vi "OOB Performance Test varaiable.vi"() -> ()   [LabVIEW 2021]
uses:
  <vilib>/Platform/TimedLoop/XDataNode/timing_clust.ctl
  <vilib>/Platform/TimedLoop/XDataNode/nitl_modes.ctl
  <vilib>/Platform/TimedLoop/XDataNode/wakeup.ctl
  CIFOutOfBand.lvclass/CIFOutOfBand.ctl
  CIFCore/Common/Typedef/Plugin Status.ctl
  CIFCore/Common/Typedef/Plugin State.ctl
  CIFCore/Common/Typedef/Timing Statistics.ctl
  CIFCore/Common/Typedef/Timing Stats Base.ctl
  CIFCore/Common/Typedef/FIFO Statistics.ctl
  CIFCore/Common/Typedef/Simple Error.ctl
  CIFCore/Common/Typedef/Monitor Doubles.ctl
  CIFCore/Common/Typedef/Monitor U64.ctl
  CIFCore/Common/Typedef/Monitor I64.ctl
  CIFOutOfBand.lvclass
  <vilib>/Platform/TimedLoop/XDataNode/XDataNode.xnode
  <vilib>/Platform/TimedLoop/XDataNode/XDNodeRunTimeDep.lvlib
  CIFCore/Common/CIFCoreCommon.lvlib
panel:
  out "avg complexwrite":dbl
  out "Max Complexwrite":dbl
  out "avg complexnote write":dbl
  out "Max Complexnote write":dbl
  out "avg complexnote":dbl
  out "Max Complexnote":dbl
  out "avg Occur":dbl
  out "Max Occur":dbl
  out "avg Notifier":dbl
  out "Max Notifier":dbl
  out "avg RTFifo":dbl
  out "Max RTFifo":dbl
  out "avg raw dvr write":dbl
  out "Max raw dvr write":dbl
  in  "stop":bool
  out "avg raw local":dbl
  out "Max raw local":dbl
  out "avg raw dvr":dbl
  out "Max raw dvr":dbl
  out "avg no conflict":dbl
  out "Max no conflict":dbl
  out "avg simple":dbl
  out "Max simple":dbl
  out "Max Complex":dbl
  out "avg complex":dbl
  out "pass":bool
  out "error out":errorcluster
  # "This test should be run on RT.  It stresses the communications by constantly creating resource contraints with the low priority sender and the high priority loop. On Windows the priority of the loops cannot be set."
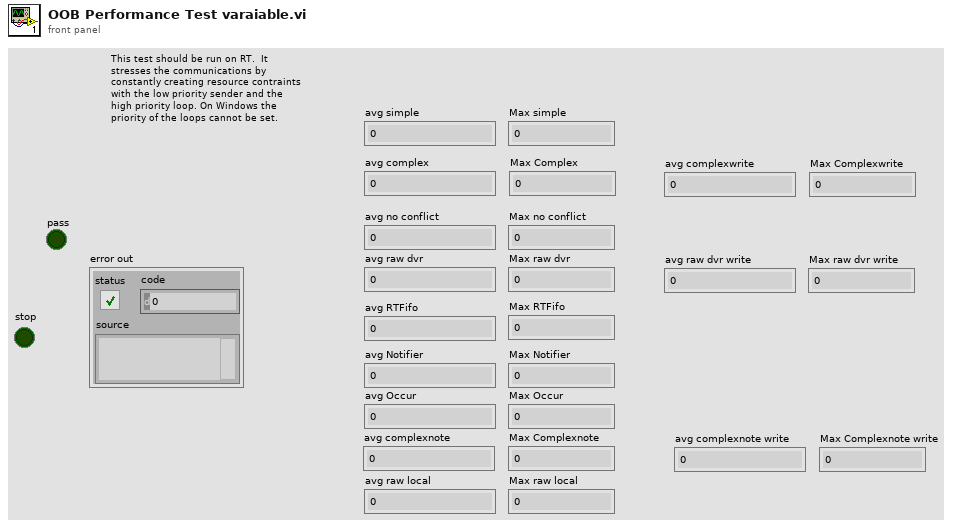
[diagram p1: front panel]
types:
  T1 = typedef "XDNodeRunTimeDep.lvlib/timing_clust.ctl" = cluster{"Expected End [f-1]":u64, "Actual End [f-1]":u64, "Finished Late? [f-1]":bool, "Expected End [i-1]":u64, "Actual End [i-1]":u64, "Finished Late? [i-1]":bool, "Expected Start [i]":u64, "Actual Start [i]":u64, "Expected Start [f]":u64, "Actual Start [f]":u64, "Source Name":string, "Structure Name":string, "Period":i64, "Deadline":i64, "Offset":i64, "Start":i64, "Priority":i32, "Timeout":i32, "Mode":T2, "Wakeup Reason":T3, "Error":errorcluster, "Source Type":string, "Secondary Source Type":string, "Global End Time":u64, "Global Start Time":u64, "Frame Duration":u64, "Iteration Duration":u64, "Assigned CPU":i32, "I/O Scan Engine Mode":u32}
  T2 = typedef "XDNodeRunTimeDep.lvlib/nitl_modes.ctl" = enum32{"No Change", "Process missed periods, maintain original phase", "Discard missed periods, maintain original phase", "Process missed periods, ignore original phase", "Discard missed periods, ignore original phase"}
  T3 = typedef "XDNodeRunTimeDep.lvlib/wakeup.ctl" = enum32{"Normal", "Aborted", "Asynchronous wakeup", "Timing source error", "Timed loop error", "Timeout"}
  T4 = cluster{"read mode":enum16{"polling", "blocking"}, "write mode":enum16{"polling", "blocking"}}
  T5 = typedef "CIFCoreCommon.lvlib/Plugin Status.ctl" = cluster{"State":T6, "Timing Statistics (us)":T7, "FIFO Statistics (us)":T9, "error":T10, "Monitor Doubles":T11, "Monitor U64":T12, "Monitor I64":T13, "Cleanup":T8, "Create":i32, "Destroy":i32}
  T6 = typedef "CIFCoreCommon.lvlib/Plugin State.ctl" = enum32{"Null", "Creating", "Listening", "Running", "CleaningUp", "Destroying"}
  T7 = typedef "CIFCoreCommon.lvlib/Timing Statistics.ctl" = cluster{"Period":T8, "Wake Error":T8, "Execute":T8, "Housekeep":T8, "Idle":T8}
  T8 = typedef "CIFCoreCommon.lvlib/Timing Stats Base.ctl" = cluster{"Max":i32, "Min":i32}
  T9 = typedef "CIFCoreCommon.lvlib/FIFO Statistics.ctl" = cluster{"From T0":T8, "From Previous Plugin":T8, "Output Error":T8}
  T10 = typedef "CIFCoreCommon.lvlib/Simple Error.ctl" = cluster{"status":bool, "code":i32}
  T11 = typedef "CIFCoreCommon.lvlib/Monitor Doubles.ctl" = cluster{"1":dbl, "2":dbl, "3":dbl, "4":dbl}
  T12 = typedef "CIFCoreCommon.lvlib/Monitor U64.ctl" = cluster{"1":u64, "2":u64, "3":u64, "4":u64}
  T13 = typedef "CIFCoreCommon.lvlib/Monitor I64.ctl" = cluster{"1":i64, "2":i64, "3":i64, "4":i64}
  T14 = cluster{"Numeric":dbl, "Array":cluster{"Numeric":dbl, "String":string, "Boolean":bool}[], "string":string, "Null array":u8[]}
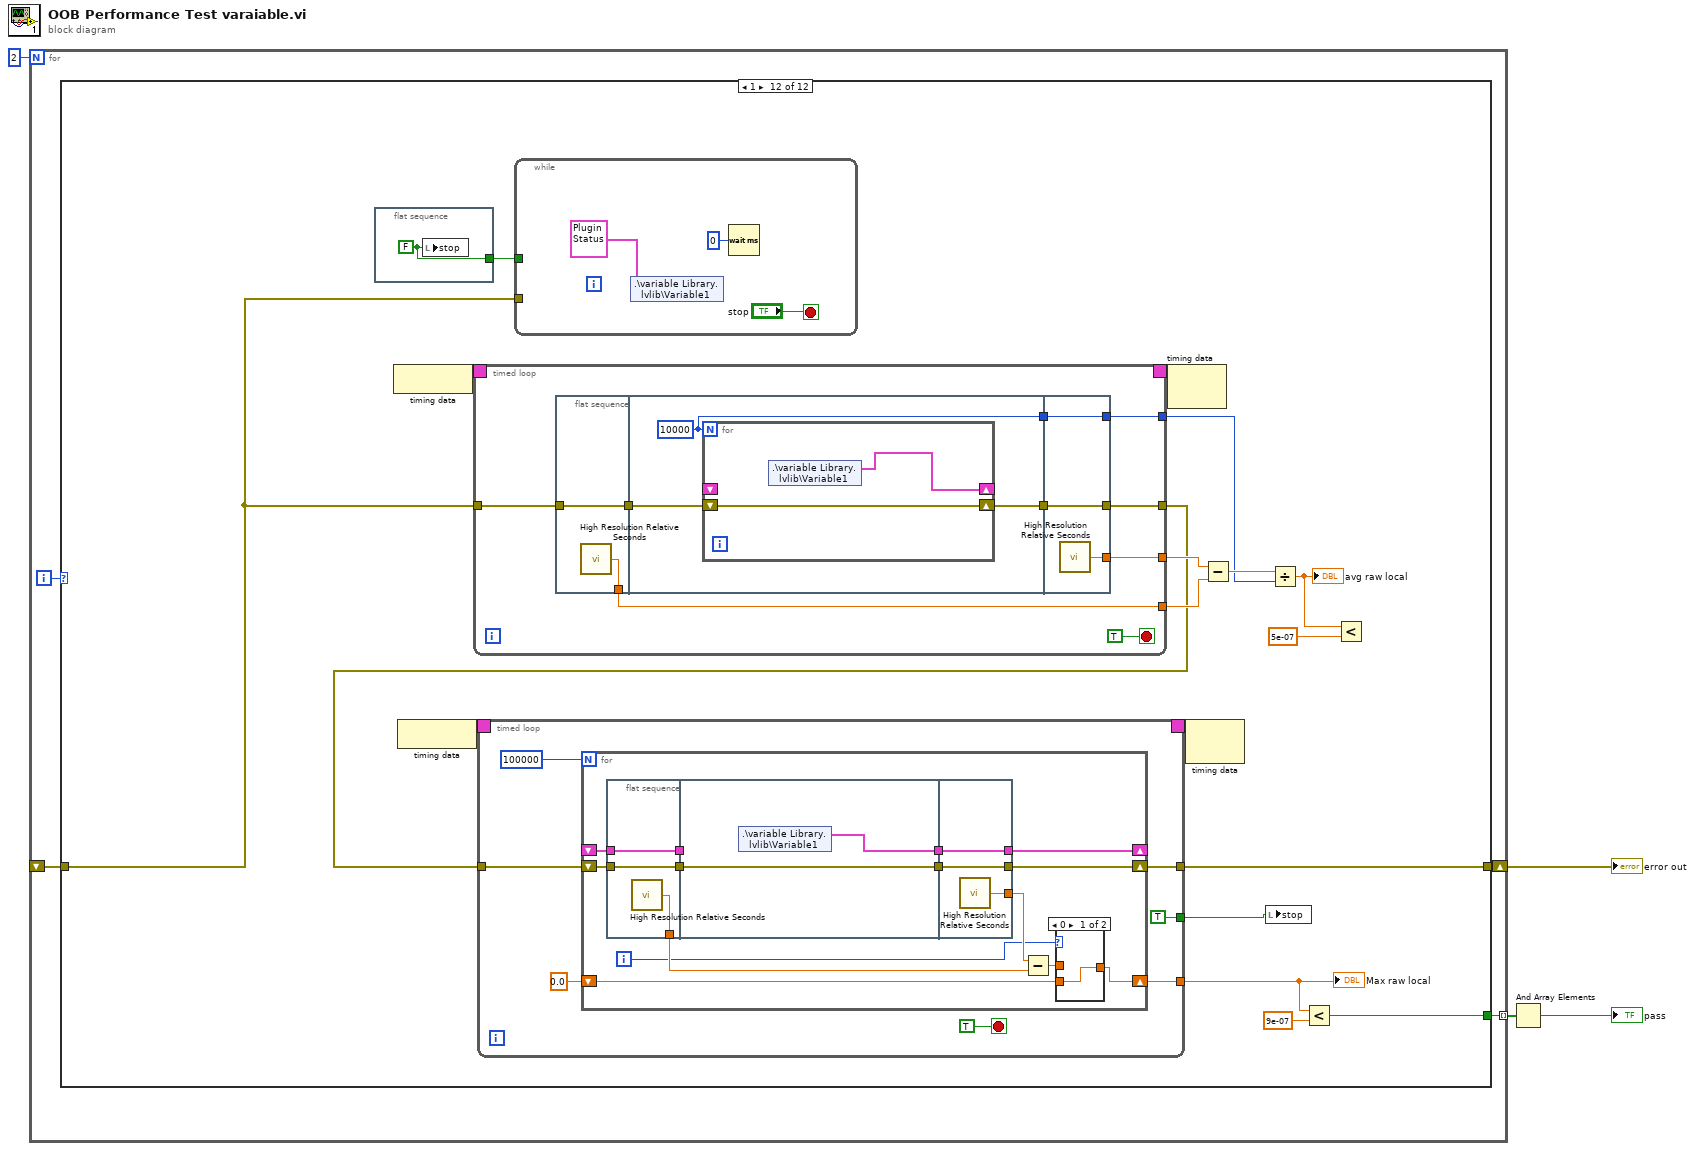
[diagram p0: block diagram]
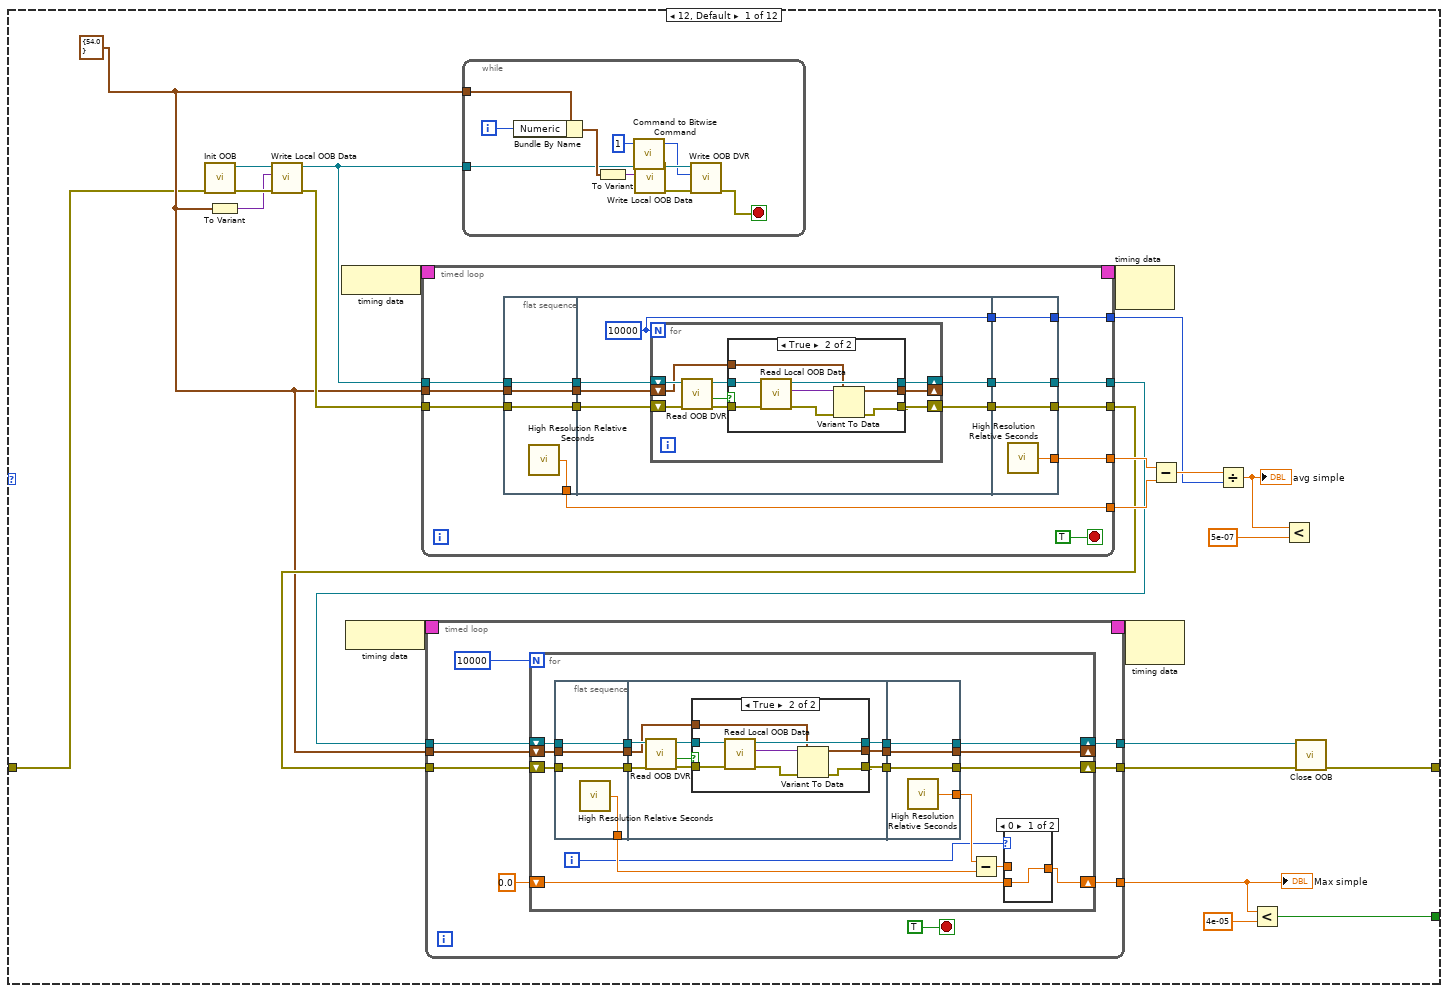
[diagram p2: hidden frame]
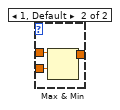
[diagram p3: hidden frame]
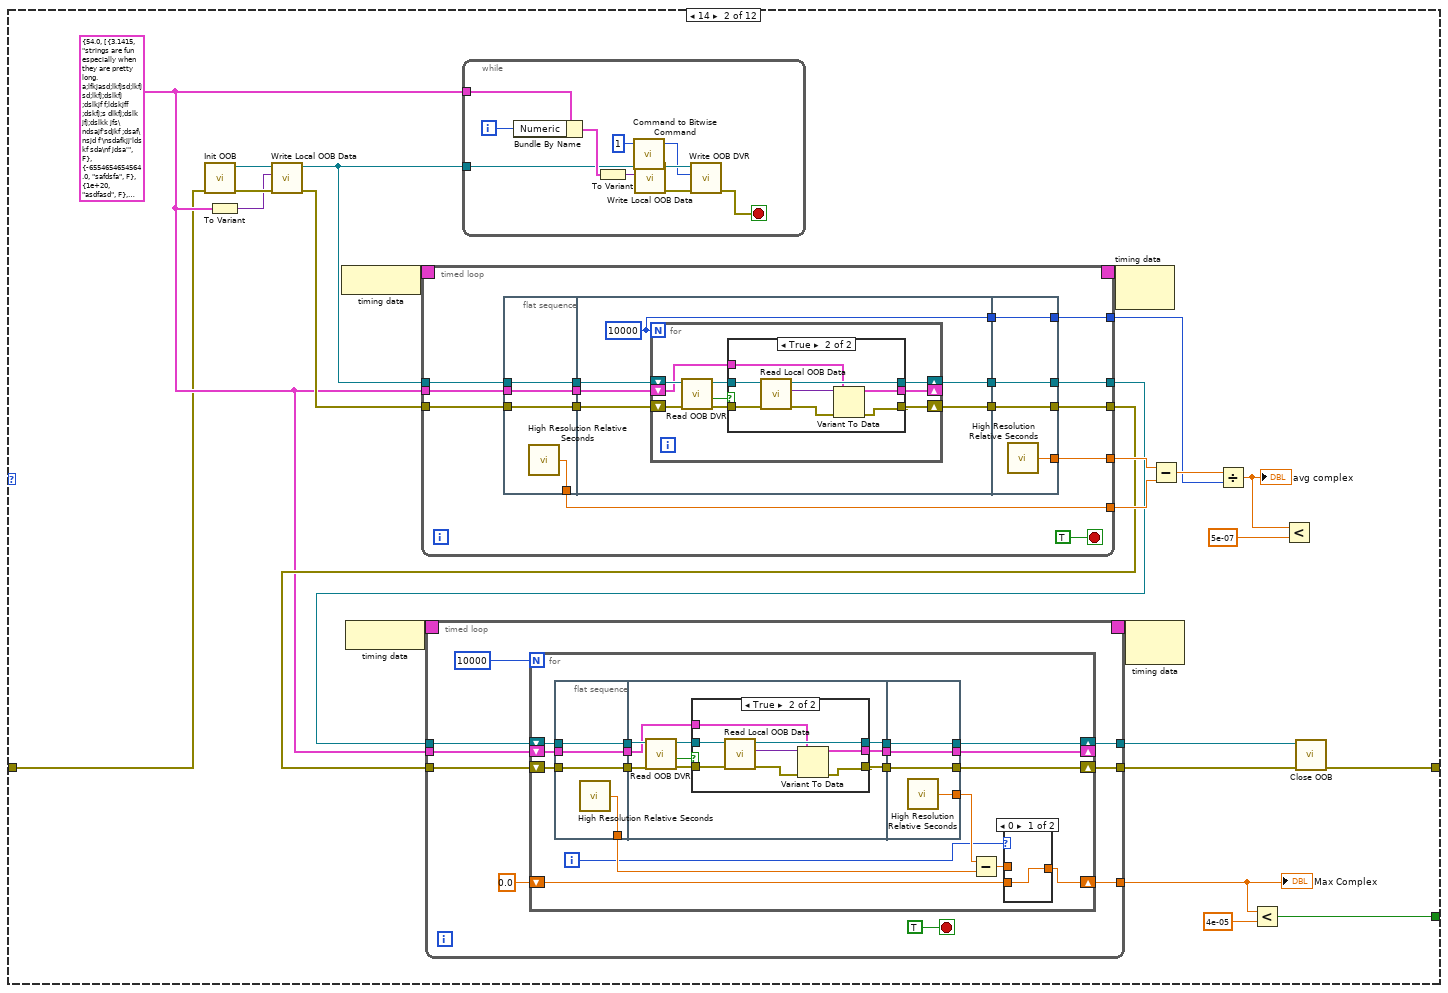
[diagram p6: hidden frame]
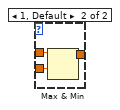
[diagram p7: hidden frame]
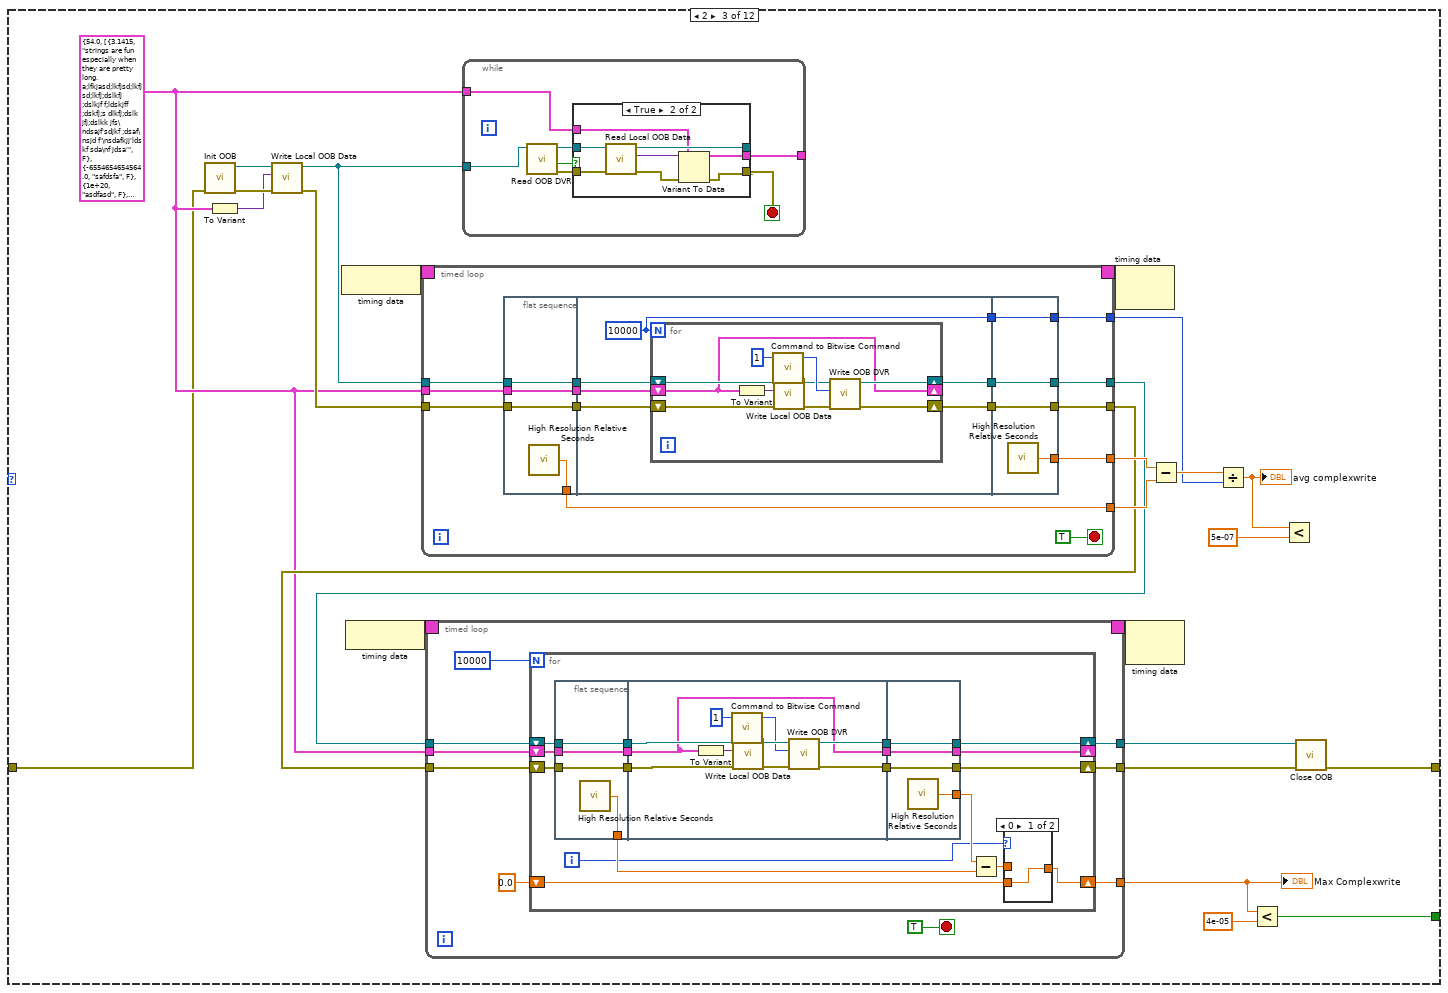
[diagram p10: hidden frame]
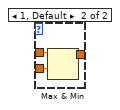
[diagram p12: hidden frame]
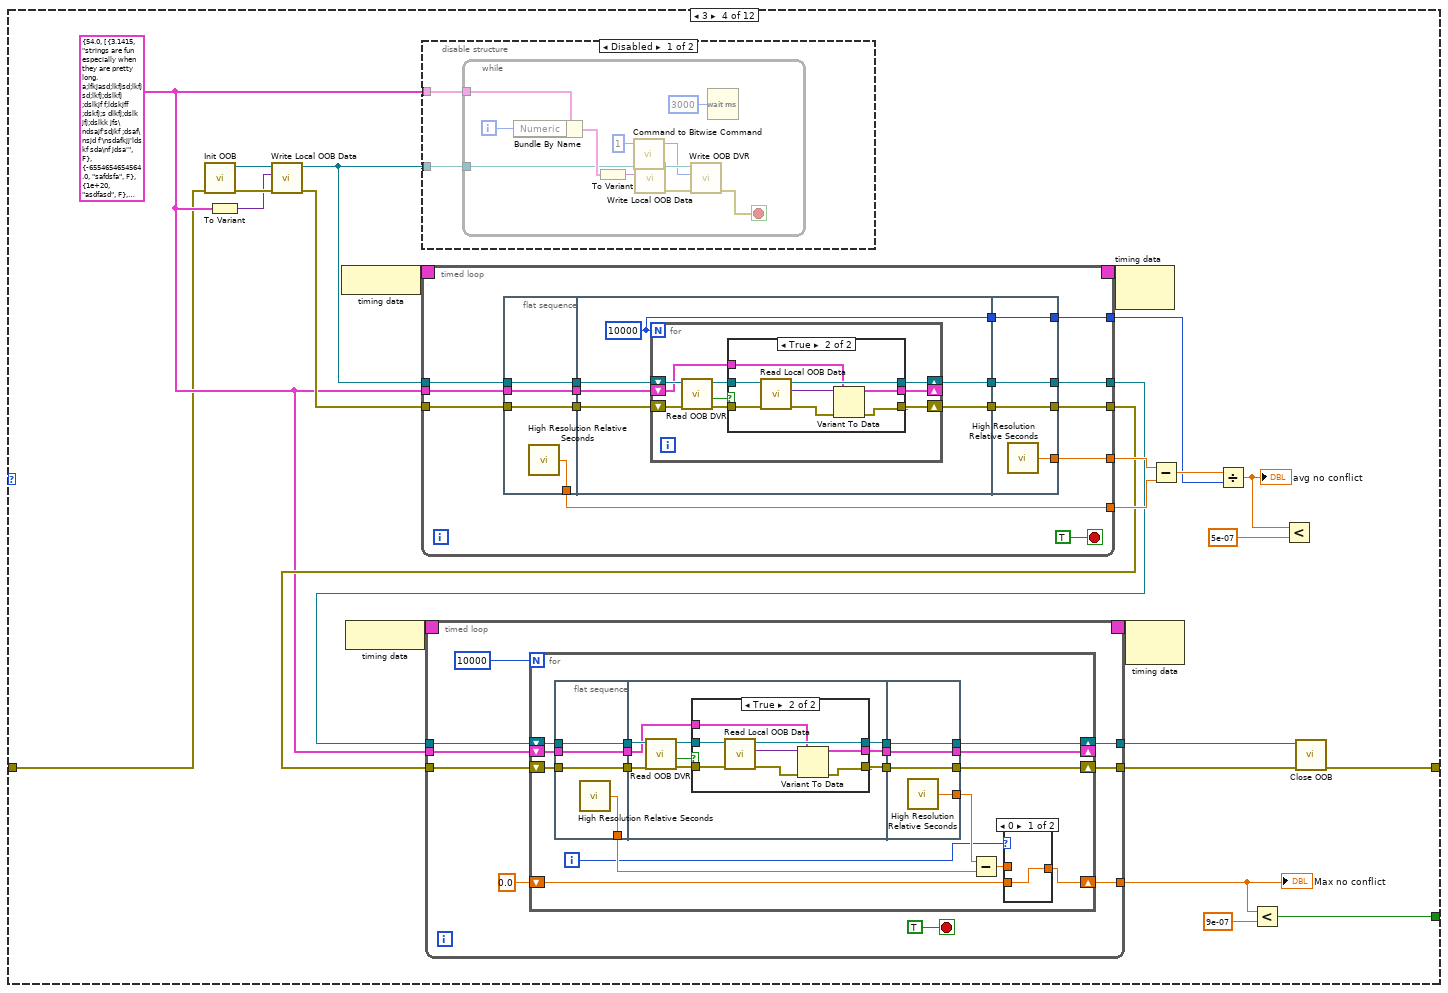
[diagram p13: hidden frame]
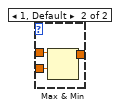
[diagram p15: hidden frame]
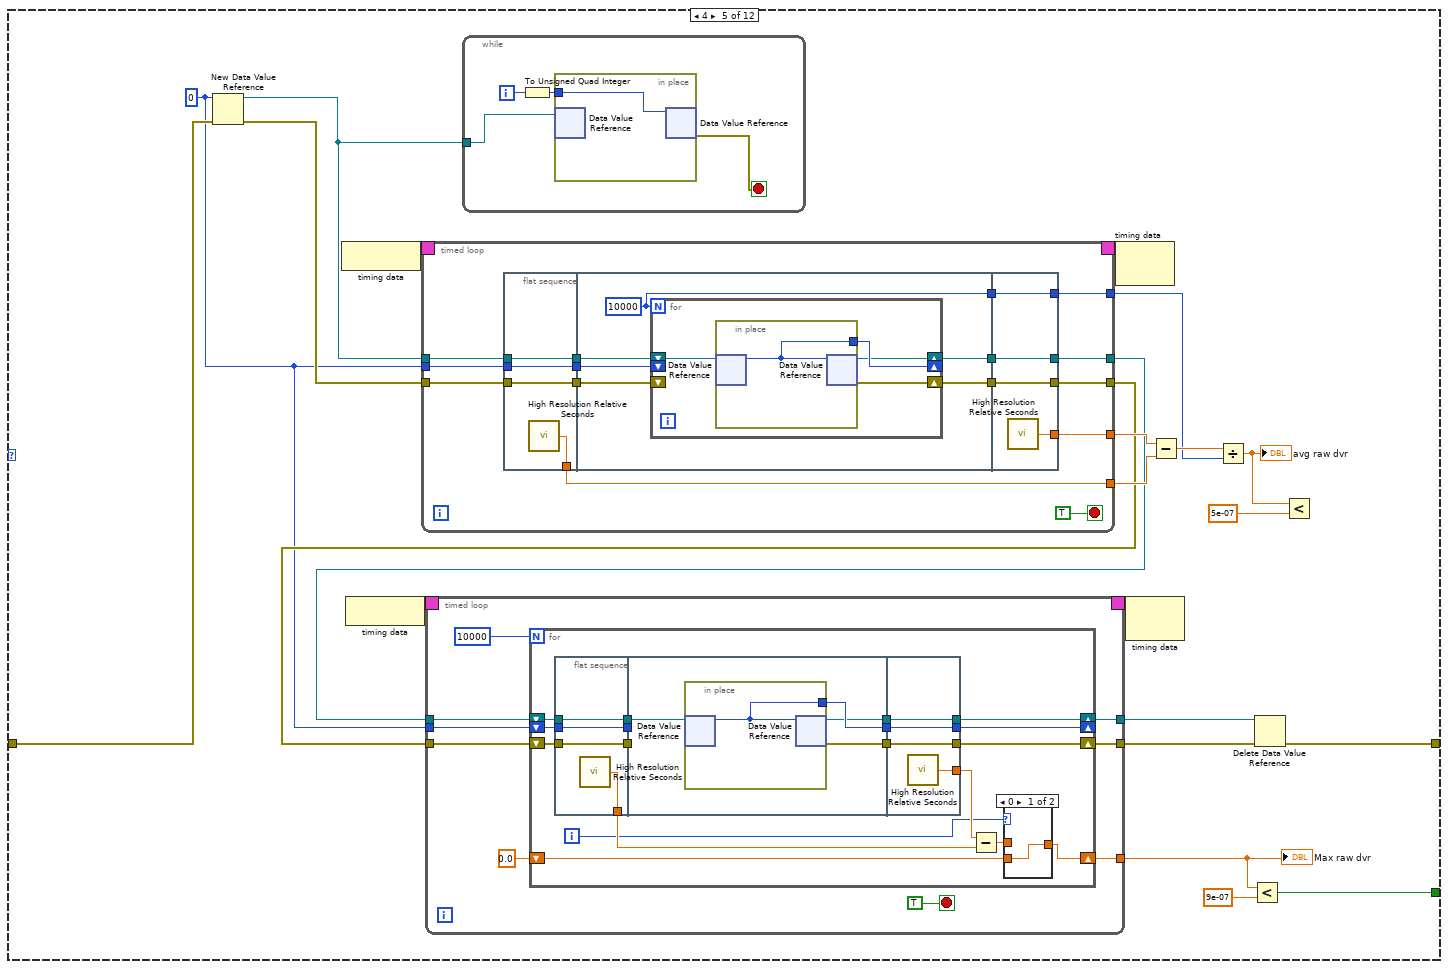
[diagram p18: hidden frame]
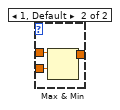
[diagram p19: hidden frame]
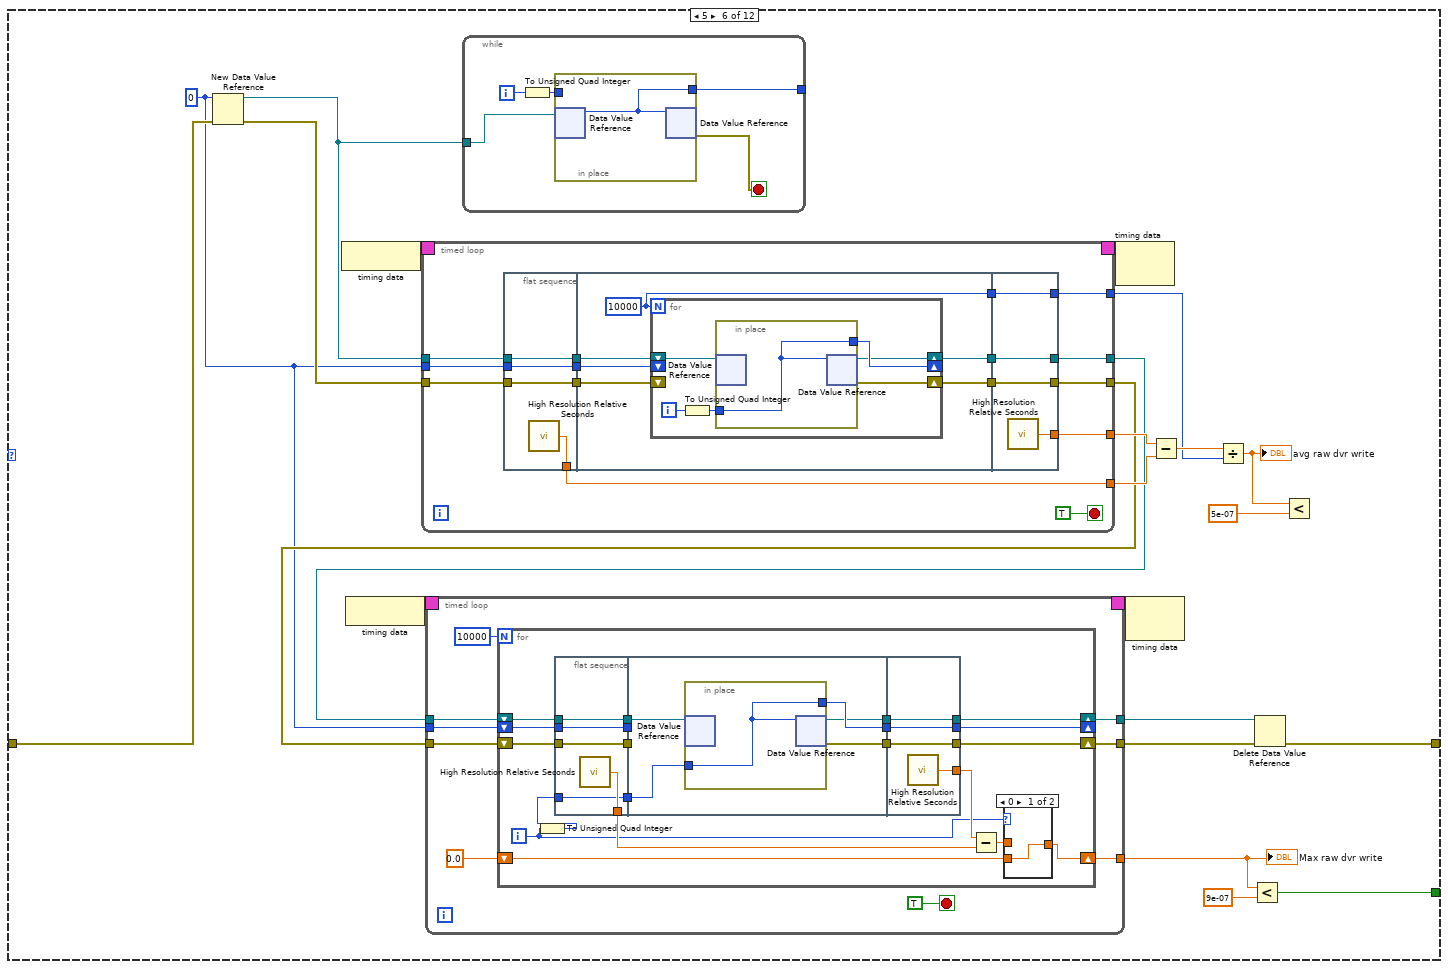
[diagram p20: hidden frame]
diagram:
  n1 = for {
    N: 2 -> [_]
    tunnel: [w8] -> w2 mode=indexing
    shift-right: [w7] -> w4
    shift-left: _ -> [w5]
    i -> [w6]
    n2 = case shown="1" w6 {
      tunnel: [w19 w168 w317 w455 w604 w717 w839 w957 w1074 w1189 w1304 w1415] -> w8
      tunnel: [w16 w165 w314 w452 w597 w710 w836 w954 w1070 w1182 w1297 w1414] -> w7
      tunnel: w5 -> [w9 w158 w307 w445 w602 w715 w833 w951 w1071 w1187 w1302 w1412]
      frame 12, Default {
        w10 = cluster{"Numeric":dbl} {"Numeric"=54.0} ("Test Config")
        n3 = call "Init OOB.vi"("error in (no error)"=w9) -> ("error out"=w15:errorcluster, "OOB out"=w13:refnum<class "CIFOutOfBand.lvclass">)  [unwired: 9 in]
        n4 = To Variant(anything=w10) -> (Variant=w14:variant)
        n5 = call "Write Local OOB Data.vi"("error in"=w15, "Local OOB Data"=w14, "OOB in"=w13) -> ("error out"=w11:errorcluster, "OOB out"=w12:refnum<class "CIFOutOfBand.lvclass">)  [unwired: 7 in]
        n6 = node-c288() -> (w33:T1)
        n7 = node-c288() -> (w31:T1)
        n8 = timed-loop {
          timing: w33 -> [_]
          timing-out: [_] -> w32
          tunnel: w12 -> [w120]
          tunnel: w11 -> [w119]
          tunnel: [w115] -> w25
          tunnel: [w113] -> w24
          tunnel: [w111] -> w29
          tunnel: [w110] -> w28
          tunnel: [w109] -> w26
          tunnel: w10 -> [w107]
          stop <- TRUE stop-if-true
          n9 = flat-sequence {
            tunnel: w119 -> [w123]
            tunnel: w120 -> [w124]
            tunnel: [w124] -> w117
            tunnel: [w123] -> w116
            tunnel: [w122] -> w110
            tunnel: w107 -> [w121]
            tunnel: [w121] -> w106
            tunnel: w117 -> [w130]
            tunnel: w116 -> [w129]
            tunnel: [w128] -> w114
            tunnel: [w127] -> w112
            tunnel: [w126] -> w108
            tunnel: w106 -> [w125]
            tunnel: [w153] -> w115
            tunnel: w114 -> [w153]
            tunnel: [w152] -> w113
            tunnel: w112 -> [w152]
            tunnel: [w151] -> w111
            tunnel: [w150] -> w109
            tunnel: w108 -> [w150]
            frame #0 {
              n10 = call <vilib>:"High Resolution Relative Seconds.vi"() -> ("relative seconds"=w122:dbl)
            }
            frame #1 {
              w126 = 10000
              n11 = for {
                N: w126 -> [_]
                shift-right: [w136] -> w128
                shift-left: w130 -> [w135]
                shift-right: [w132] -> w127
                shift-left: w129 -> [w133]
                shift-right: [w131] -> _
                shift-left: w125 -> [w134]
                n12 = call "Read OOB DVR.vi"("error in"=w133, "OOB in"=w135) -> ("error out"=w137:errorcluster, "New Commands"=w139:bool, "OOB out"=w138:refnum<class "CIFOutOfBand.lvclass">)  [unwired: 6 in, 1 out]
                n13 = case shown="True" w139 {
                  tunnel: w138 -> [w140 w149]
                  tunnel: w137 -> [w141 w148]
                  tunnel: [w140 w146] -> w136
                  tunnel: w134 -> [_ w144]
                  tunnel: [_ w142] -> w131
                  tunnel: [w141 w143] -> w132
                  frame False {
                  }
                  frame True {
                    n14 = call "Read Local OOB Data.vi"("error in"=w148, "OOB in"=w149) -> ("error out"=w147:errorcluster, "Local OOB Data"=w145:variant, "OOB out"=w146:refnum<class "CIFOutOfBand.lvclass">)  [unwired: 7 in]
                    n15 = Variant To Data(error in=w147, type=w144, Variant=w145) -> (data=w142:cluster{"Numeric":dbl}, error out=w143:errorcluster)
                  }
                }
              }
            }
            frame #2 {
              n16 = call <vilib>:"High Resolution Relative Seconds.vi"() -> ("relative seconds"=w151:dbl)
            }
          }
        }
        n17 = timed-loop {
          timing: w31 -> [_]
          timing-out: [_] -> w30
          tunnel: w25 -> [w52]
          tunnel: w24 -> [w51]
          tunnel: [w49] -> w18
          tunnel: [w48] -> w17
          tunnel: w10 -> [w47]
          tunnel: [w44] -> w21
          stop <- TRUE stop-if-true
          n18 = for {
            N: 10000 -> [_]
            shift-right: [w64] -> w49
            shift-left: w52 -> [w66]
            shift-right: [w63] -> w48
            shift-left: w51 -> [w65]
            shift-right: [w57] -> w44
            shift-left: 0.0 -> [w58]
            shift-right: [w56] -> _
            shift-left: w47 -> [w62]
            i -> [w54]
            n19 = flat-sequence {
              tunnel: w65 -> [w77]
              tunnel: w66 -> [w78]
              tunnel: [w78] -> w70
              tunnel: [w77] -> w69
              tunnel: [w76] -> w60
              tunnel: w62 -> [w75]
              tunnel: [w75] -> w68
              tunnel: w70 -> [w84]
              tunnel: w69 -> [w82]
              tunnel: [w81] -> w67
              tunnel: w68 -> [w83]
              tunnel: [w80] -> w55
              tunnel: [w79] -> w53
              tunnel: [w101] -> w64
              tunnel: w67 -> [w101]
              tunnel: [w100] -> w63
              tunnel: [w99] -> w61
              tunnel: [w98] -> w56
              tunnel: w55 -> [w98]
              tunnel: w53 -> [w100]
              frame #0 {
                n20 = call <vilib>:"High Resolution Relative Seconds.vi"() -> ("relative seconds"=w76:dbl)
              }
              frame #1 {
                n21 = call "Read OOB DVR.vi"("error in"=w82, "OOB in"=w84) -> ("error out"=w87:errorcluster, "New Commands"=w85:bool, "OOB out"=w86:refnum<class "CIFOutOfBand.lvclass">)  [unwired: 6 in, 1 out]
                n22 = case shown="True" w85 {
                  tunnel: w86 -> [w88 w97]
                  tunnel: w87 -> [w89 w96]
                  tunnel: [w88 w94] -> w81
                  tunnel: w83 -> [_ w92]
                  tunnel: [_ w90] -> w80
                  tunnel: [w89 w91] -> w79
                  frame False {
                  }
                  frame True {
                    n23 = call "Read Local OOB Data.vi"("error in"=w96, "OOB in"=w97) -> ("error out"=w95:errorcluster, "Local OOB Data"=w93:variant, "OOB out"=w94:refnum<class "CIFOutOfBand.lvclass">)  [unwired: 7 in]
                    n24 = Variant To Data(error in=w95, type=w92, Variant=w93) -> (data=w90:cluster{"Numeric":dbl}, error out=w91:errorcluster)
                  }
                }
              }
              frame #2 {
                n25 = call <vilib>:"High Resolution Relative Seconds.vi"() -> ("relative seconds"=w99:dbl)
              }
            }
            n26 = Subtract(x=w61, y=w60) -> (x-y=w59:dbl)
            n27 = case shown="0" w54 {
              tunnel: w59 -> [_ w74]
              tunnel: w58 -> [w71 w73]
              tunnel: [w71 w72] -> w57
              frame 0 {
              }
              frame 1, Default {
                n28 = Max & Min(x=w74, y=w73) -> (max(x,y)=w72:dbl)  [unwired: 1 out]
              }
            }
          }
        }
        "Max simple" <- w21
        n29 = while {
          tunnel: w12 -> [w35]
          tunnel: w10 -> [w42]
          i -> [w43]
          stop <- w34 stop-if-true
          n30 = Bundle By Name(cluster=w42, "Numeric"=w43) -> (w36:cluster{"Numeric":dbl})
          n31 = To Variant(anything=w36) -> (Variant=w38:variant)
          n32 = call "Command to Bitwise Command.vi"("OOB Command"=u8 1) -> ("bit command"=w37:u64)  [unwired: 3 in]
          n33 = call "Write Local OOB Data.vi"("Local OOB Data"=w38, "OOB in"=w35) -> ("error out"=w39:errorcluster, "OOB out"=w40:refnum<class "CIFOutOfBand.lvclass">)  [unwired: 8 in]
          n34 = call "Write OOB DVR.vi"("error in"=w39, "Commands (bitwise)"=w37, "OOB in"=w40) -> ("error out"=w34:errorcluster)  [unwired: 7 in, 1 out]
        }
        n35 = node-c288(w32) -> ()  [unwired: 1 out]
        n36 = node-c288(w30) -> ()  [unwired: 1 out]
        n37 = Subtract(x=w29, y=w28) -> (x-y=w27:dbl)
        n38 = Divide(x=w27, y=w26) -> (x/y=w23:dbl)
        "avg simple" <- w23
        n39 = Less?(x=w21, y=4e-05) -> (x < y?=w19:bool)
        n40 = Less?(x=w23, y=5e-07) -> ()  [unwired: 1 out]
        n41 = call "Close OOB.vi"("error in"=w17, "OOB in"=w18) -> ("error out"=w16:errorcluster)  [unwired: 9 in]
      }
      frame 14 {
        w159 = T14 {"Numeric"=54.0, "Array"=[{"Numeric"=3.1415, "String"="strings are fun especially when they are pretty long. a;lfkjasd;lkfjsd;lkfjsd;lkfj;dslkfj ;dslkjf f;ldskjff ;dskfj;s dlkfj;dslk jfj;dslkk jfs\ndsajf'sdjkf ;dsaf\nsjd f'\nsdafkjj'lds kf sda\nf jdsa'", "Boolean"=FALSE}, {"Numeric"=-6554654654564.0, "String"="safdsfa", "Boolean"=FALSE}, {"Numeric"=1e+20, "String"="asdfasd", "Boolean"=FALSE}, {"Numeric"=2.0, "String"="afd", "Boolean"=TRUE}, {"Numeric"=12.34, "String"="data", "Boolean"=FALSE}], "string"="strings", "Null array"=[0]} ("Test Config")
        n42 = call "Init OOB.vi"("error in (no error)"=w158) -> ("error out"=w164:errorcluster, "OOB out"=w162:refnum<class "CIFOutOfBand.lvclass">)  [unwired: 9 in]
        n43 = To Variant(anything=w159) -> (Variant=w163:variant)
        n44 = call "Write Local OOB Data.vi"("error in"=w164, "Local OOB Data"=w163, "OOB in"=w162) -> ("error out"=w160:errorcluster, "OOB out"=w161:refnum<class "CIFOutOfBand.lvclass">)  [unwired: 7 in]
        n45 = node-c288() -> (w182:T1)
        n46 = node-c288() -> (w180:T1)
        n47 = timed-loop {
          timing: w182 -> [_]
          timing-out: [_] -> w181
          tunnel: w161 -> [w269]
          tunnel: w160 -> [w268]
          tunnel: [w264] -> w174
          tunnel: [w262] -> w173
          tunnel: [w260] -> w178
          tunnel: [w259] -> w177
          tunnel: [w258] -> w175
          tunnel: w159 -> [w256]
          stop <- TRUE stop-if-true
          n48 = flat-sequence {
            tunnel: w268 -> [w272]
            tunnel: w269 -> [w273]
            tunnel: [w273] -> w266
            tunnel: [w272] -> w265
            tunnel: [w271] -> w259
            tunnel: w256 -> [w270]
            tunnel: [w270] -> w255
            tunnel: w266 -> [w279]
            tunnel: w265 -> [w278]
            tunnel: [w277] -> w263
            tunnel: [w276] -> w261
            tunnel: [w275] -> w257
            tunnel: w255 -> [w274]
            tunnel: [w302] -> w264
            tunnel: w263 -> [w302]
            tunnel: [w301] -> w262
            tunnel: w261 -> [w301]
            tunnel: [w300] -> w260
            tunnel: [w299] -> w258
            tunnel: w257 -> [w299]
            frame #0 {
              n49 = call <vilib>:"High Resolution Relative Seconds.vi"() -> ("relative seconds"=w271:dbl)
            }
            frame #1 {
              w275 = 10000
              n50 = for {
                N: w275 -> [_]
                shift-right: [w285] -> w277
                shift-left: w279 -> [w284]
                shift-right: [w281] -> w276
                shift-left: w278 -> [w282]
                shift-right: [w280] -> _
                shift-left: w274 -> [w283]
                n51 = call "Read OOB DVR.vi"("error in"=w282, "OOB in"=w284) -> ("error out"=w286:errorcluster, "New Commands"=w288:bool, "OOB out"=w287:refnum<class "CIFOutOfBand.lvclass">)  [unwired: 6 in, 1 out]
                n52 = case shown="True" w288 {
                  tunnel: w287 -> [w289 w298]
                  tunnel: w286 -> [w290 w297]
                  tunnel: [w289 w295] -> w285
                  tunnel: w283 -> [_ w293]
                  tunnel: [_ w291] -> w280
                  tunnel: [w290 w292] -> w281
                  frame False {
                  }
                  frame True {
                    n53 = call "Read Local OOB Data.vi"("error in"=w297, "OOB in"=w298) -> ("error out"=w296:errorcluster, "Local OOB Data"=w294:variant, "OOB out"=w295:refnum<class "CIFOutOfBand.lvclass">)  [unwired: 7 in]
                    n54 = Variant To Data(error in=w296, type=w293, Variant=w294) -> (data=w291:T14, error out=w292:errorcluster)
                  }
                }
              }
            }
            frame #2 {
              n55 = call <vilib>:"High Resolution Relative Seconds.vi"() -> ("relative seconds"=w300:dbl)
            }
          }
        }
        n56 = timed-loop {
          timing: w180 -> [_]
          timing-out: [_] -> w179
          tunnel: w174 -> [w201]
          tunnel: w173 -> [w200]
          tunnel: [w198] -> w167
          tunnel: [w197] -> w166
          tunnel: w159 -> [w196]
          tunnel: [w193] -> w170
          stop <- TRUE stop-if-true
          n57 = for {
            N: 10000 -> [_]
            shift-right: [w213] -> w198
            shift-left: w201 -> [w215]
            shift-right: [w212] -> w197
            shift-left: w200 -> [w214]
            shift-right: [w206] -> w193
            shift-left: 0.0 -> [w207]
            shift-right: [w205] -> _
            shift-left: w196 -> [w211]
            i -> [w203]
            n58 = flat-sequence {
              tunnel: w214 -> [w226]
              tunnel: w215 -> [w227]
              tunnel: [w227] -> w219
              tunnel: [w226] -> w218
              tunnel: [w225] -> w209
              tunnel: w211 -> [w224]
              tunnel: [w224] -> w217
              tunnel: w219 -> [w233]
              tunnel: w218 -> [w231]
              tunnel: [w230] -> w216
              tunnel: w217 -> [w232]
              tunnel: [w229] -> w204
              tunnel: [w228] -> w202
              tunnel: [w250] -> w213
              tunnel: w216 -> [w250]
              tunnel: [w249] -> w212
              tunnel: [w248] -> w210
              tunnel: [w247] -> w205
              tunnel: w204 -> [w247]
              tunnel: w202 -> [w249]
              frame #0 {
                n59 = call <vilib>:"High Resolution Relative Seconds.vi"() -> ("relative seconds"=w225:dbl)
              }
              frame #1 {
                n60 = call "Read OOB DVR.vi"("error in"=w231, "OOB in"=w233) -> ("error out"=w236:errorcluster, "New Commands"=w234:bool, "OOB out"=w235:refnum<class "CIFOutOfBand.lvclass">)  [unwired: 6 in, 1 out]
                n61 = case shown="True" w234 {
                  tunnel: w235 -> [w237 w246]
                  tunnel: w236 -> [w238 w245]
                  tunnel: [w237 w243] -> w230
                  tunnel: w232 -> [_ w241]
                  tunnel: [_ w239] -> w229
                  tunnel: [w238 w240] -> w228
                  frame False {
                  }
                  frame True {
                    n62 = call "Read Local OOB Data.vi"("error in"=w245, "OOB in"=w246) -> ("error out"=w244:errorcluster, "Local OOB Data"=w242:variant, "OOB out"=w243:refnum<class "CIFOutOfBand.lvclass">)  [unwired: 7 in]
                    n63 = Variant To Data(error in=w244, type=w241, Variant=w242) -> (data=w239:T14, error out=w240:errorcluster)
                  }
                }
              }
              frame #2 {
                n64 = call <vilib>:"High Resolution Relative Seconds.vi"() -> ("relative seconds"=w248:dbl)
              }
            }
            n65 = Subtract(x=w210, y=w209) -> (x-y=w208:dbl)
            n66 = case shown="0" w203 {
              tunnel: w208 -> [_ w223]
              tunnel: w207 -> [w220 w222]
              tunnel: [w220 w221] -> w206
              frame 0 {
              }
              frame 1, Default {
                n67 = Max & Min(x=w223, y=w222) -> (max(x,y)=w221:dbl)  [unwired: 1 out]
              }
            }
          }
        }
        "Max Complex" <- w170
        n68 = while {
          tunnel: w161 -> [w184]
          tunnel: w159 -> [w191]
          i -> [w192]
          stop <- w183 stop-if-true
          n69 = Bundle By Name(cluster=w191, "Numeric"=w192) -> (w185:T14)
          n70 = To Variant(anything=w185) -> (Variant=w187:variant)
          n71 = call "Command to Bitwise Command.vi"("OOB Command"=u8 1) -> ("bit command"=w186:u64)  [unwired: 3 in]
          n72 = call "Write Local OOB Data.vi"("Local OOB Data"=w187, "OOB in"=w184) -> ("error out"=w188:errorcluster, "OOB out"=w189:refnum<class "CIFOutOfBand.lvclass">)  [unwired: 8 in]
          n73 = call "Write OOB DVR.vi"("error in"=w188, "Commands (bitwise)"=w186, "OOB in"=w189) -> ("error out"=w183:errorcluster)  [unwired: 7 in, 1 out]
        }
        n74 = node-c288(w181) -> ()  [unwired: 1 out]
        n75 = node-c288(w179) -> ()  [unwired: 1 out]
        n76 = Subtract(x=w178, y=w177) -> (x-y=w176:dbl)
        n77 = Divide(x=w176, y=w175) -> (x/y=w172:dbl)
        "avg complex" <- w172
        n78 = Less?(x=w170, y=4e-05) -> (x < y?=w168:bool)
        n79 = Less?(x=w172, y=5e-07) -> ()  [unwired: 1 out]
        n80 = call "Close OOB.vi"("error in"=w166, "OOB in"=w167) -> ("error out"=w165:errorcluster)  [unwired: 9 in]
      }
      frame 2 {
        w308 = T14 {"Numeric"=54.0, "Array"=[{"Numeric"=3.1415, "String"="strings are fun especially when they are pretty long. a;lfkjasd;lkfjsd;lkfjsd;lkfj;dslkfj ;dslkjf f;ldskjff ;dskfj;s dlkfj;dslk jfj;dslkk jfs\ndsajf'sdjkf ;dsaf\nsjd f'\nsdafkjj'lds kf sda\nf jdsa'", "Boolean"=FALSE}, {"Numeric"=-6554654654564.0, "String"="safdsfa", "Boolean"=FALSE}, {"Numeric"=1e+20, "String"="asdfasd", "Boolean"=FALSE}, {"Numeric"=2.0, "String"="afd", "Boolean"=TRUE}, {"Numeric"=12.34, "String"="data", "Boolean"=FALSE}], "string"="strings", "Null array"=[0]} ("Test Config")
        n81 = call "Init OOB.vi"("error in (no error)"=w307) -> ("error out"=w313:errorcluster, "OOB out"=w311:refnum<class "CIFOutOfBand.lvclass">)  [unwired: 9 in]
        n82 = To Variant(anything=w308) -> (Variant=w312:variant)
        n83 = call "Write Local OOB Data.vi"("error in"=w313, "Local OOB Data"=w312, "OOB in"=w311) -> ("error out"=w309:errorcluster, "OOB out"=w310:refnum<class "CIFOutOfBand.lvclass">)  [unwired: 7 in]
        n84 = node-c288() -> (w331:T1)
        n85 = node-c288() -> (w329:T1)
        n86 = timed-loop {
          timing: w331 -> [_]
          timing-out: [_] -> w330
          tunnel: w310 -> [w416]
          tunnel: w309 -> [w415]
          tunnel: [w411] -> w323
          tunnel: [w409] -> w322
          tunnel: [w407] -> w327
          tunnel: [w406] -> w326
          tunnel: [w405] -> w324
          tunnel: w308 -> [w403]
          stop <- TRUE stop-if-true
          n87 = flat-sequence {
            tunnel: w415 -> [w419]
            tunnel: w416 -> [w420]
            tunnel: [w420] -> w413
            tunnel: [w419] -> w412
            tunnel: [w418] -> w406
            tunnel: w403 -> [w417]
            tunnel: [w417] -> w402
            tunnel: w413 -> [w426]
            tunnel: w412 -> [w425]
            tunnel: [w424] -> w410
            tunnel: [w423] -> w408
            tunnel: [w422] -> w404
            tunnel: w402 -> [w421]
            tunnel: [w440] -> w411
            tunnel: w410 -> [w440]
            tunnel: [w439] -> w409
            tunnel: w408 -> [w439]
            tunnel: [w438] -> w407
            tunnel: [w437] -> w405
            tunnel: w404 -> [w437]
            frame #0 {
              n88 = call <vilib>:"High Resolution Relative Seconds.vi"() -> ("relative seconds"=w418:dbl)
            }
            frame #1 {
              w422 = 10000
              n89 = for {
                N: w422 -> [_]
                shift-right: [w428] -> w424
                shift-left: w426 -> [w429]
                shift-right: [w430] -> w423
                shift-left: w425 -> [w431]
                shift-right: [w427] -> _
                shift-left: w421 -> [w427]
                n90 = To Variant(anything=w427) -> (Variant=w435:variant)
                n91 = call "Command to Bitwise Command.vi"("OOB Command"=u8 1) -> ("bit command"=w436:u64)  [unwired: 3 in]
                n92 = call "Write Local OOB Data.vi"("error in"=w431, "Local OOB Data"=w435, "OOB in"=w429) -> ("error out"=w434:errorcluster, "OOB out"=w433:refnum<class "CIFOutOfBand.lvclass">)  [unwired: 7 in]
                n93 = call "Write OOB DVR.vi"("error in"=w434, "Commands (bitwise)"=w436, "OOB in"=w433) -> ("error out"=w430:errorcluster, "OOB out"=w428:refnum<class "CIFOutOfBand.lvclass">)  [unwired: 7 in]
              }
            }
            frame #2 {
              n94 = call <vilib>:"High Resolution Relative Seconds.vi"() -> ("relative seconds"=w438:dbl)
            }
          }
        }
        n95 = timed-loop {
          timing: w329 -> [_]
          timing-out: [_] -> w328
          tunnel: w323 -> [w357]
          tunnel: w322 -> [w356]
          tunnel: [w354] -> w316
          tunnel: [w353] -> w315
          tunnel: w308 -> [w352]
          tunnel: [w349] -> w319
          stop <- TRUE stop-if-true
          n96 = for {
            N: 10000 -> [_]
            shift-right: [w369] -> w354
            shift-left: w357 -> [w371]
            shift-right: [w368] -> w353
            shift-left: w356 -> [w370]
            shift-right: [w362] -> w349
            shift-left: 0.0 -> [w363]
            shift-right: [w361] -> _
            shift-left: w352 -> [w367]
            i -> [w360]
            n97 = flat-sequence {
              tunnel: w370 -> [w382]
              tunnel: w371 -> [w383]
              tunnel: [w383] -> w375
              tunnel: [w382] -> w374
              tunnel: [w381] -> w365
              tunnel: w367 -> [w380]
              tunnel: [w380] -> w373
              tunnel: w375 -> [w387]
              tunnel: w374 -> [w388]
              tunnel: [w385] -> w372
              tunnel: w373 -> [w384]
              tunnel: [w386] -> w359
              tunnel: [w384] -> w358
              tunnel: [w397] -> w369
              tunnel: w372 -> [w397]
              tunnel: [w396] -> w368
              tunnel: [w395] -> w366
              tunnel: [w394] -> w361
              tunnel: w359 -> [w396]
              tunnel: w358 -> [w394]
              frame #0 {
                n98 = call <vilib>:"High Resolution Relative Seconds.vi"() -> ("relative seconds"=w381:dbl)
              }
              frame #1 {
                n99 = To Variant(anything=w384) -> (Variant=w390:variant)
                n100 = call "Command to Bitwise Command.vi"("OOB Command"=u8 1) -> ("bit command"=w389:u64)  [unwired: 3 in]
                n101 = call "Write Local OOB Data.vi"("error in"=w388, "Local OOB Data"=w390, "OOB in"=w387) -> ("error out"=w391:errorcluster, "OOB out"=w392:refnum<class "CIFOutOfBand.lvclass">)  [unwired: 7 in]
                n102 = call "Write OOB DVR.vi"("error in"=w391, "Commands (bitwise)"=w389, "OOB in"=w392) -> ("error out"=w386:errorcluster, "OOB out"=w385:refnum<class "CIFOutOfBand.lvclass">)  [unwired: 7 in]
              }
              frame #2 {
                n103 = call <vilib>:"High Resolution Relative Seconds.vi"() -> ("relative seconds"=w395:dbl)
              }
            }
            n104 = Subtract(x=w366, y=w365) -> (x-y=w364:dbl)
            n105 = case shown="0" w360 {
              tunnel: w364 -> [_ w379]
              tunnel: w363 -> [w376 w378]
              tunnel: [w376 w377] -> w362
              frame 0 {
              }
              frame 1, Default {
                n106 = Max & Min(x=w379, y=w378) -> (max(x,y)=w377:dbl)  [unwired: 1 out]
              }
            }
          }
        }
        "Max Complexwrite" <- w319
        n107 = while {
          tunnel: w310 -> [w333]
          tunnel: w308 -> [w334]
          tunnel: [w332] -> _
          stop <- w335 stop-if-true
          n108 = call "Read OOB DVR.vi"("OOB in"=w333) -> ("error out"=w336:errorcluster, "New Commands"=w338:bool, "OOB out"=w337:refnum<class "CIFOutOfBand.lvclass">)  [unwired: 7 in, 1 out]
          n109 = case shown="True" w338 {
            tunnel: w337 -> [w339 w348]
            tunnel: w336 -> [w340 w347]
            tunnel: [w339 w345] -> _
            tunnel: w334 -> [_ w343]
            tunnel: [_ w341] -> w332
            tunnel: [w340 w342] -> w335
            frame False {
            }
            frame True {
              n110 = call "Read Local OOB Data.vi"("error in"=w347, "OOB in"=w348) -> ("error out"=w346:errorcluster, "Local OOB Data"=w344:variant, "OOB out"=w345:refnum<class "CIFOutOfBand.lvclass">)  [unwired: 7 in]
              n111 = Variant To Data(error in=w346, type=w343, Variant=w344) -> (data=w341:T14, error out=w342:errorcluster)
            }
          }
        }
        n112 = node-c288(w330) -> ()  [unwired: 1 out]
        n113 = node-c288(w328) -> ()  [unwired: 1 out]
        n114 = Subtract(x=w327, y=w326) -> (x-y=w325:dbl)
        n115 = Divide(x=w325, y=w324) -> (x/y=w321:dbl)
        "avg complexwrite" <- w321
        n116 = Less?(x=w319, y=4e-05) -> (x < y?=w317:bool)
        n117 = Less?(x=w321, y=5e-07) -> ()  [unwired: 1 out]
        n118 = call "Close OOB.vi"("error in"=w315, "OOB in"=w316) -> ("error out"=w314:errorcluster)  [unwired: 9 in]
      }
      frame 3 {
        w446 = T14 {"Numeric"=54.0, "Array"=[{"Numeric"=3.1415, "String"="strings are fun especially when they are pretty long. a;lfkjasd;lkfjsd;lkfjsd;lkfj;dslkfj ;dslkjf f;ldskjff ;dskfj;s dlkfj;dslk jfj;dslkk jfs\ndsajf'sdjkf ;dsaf\nsjd f'\nsdafkjj'lds kf sda\nf jdsa'", "Boolean"=FALSE}, {"Numeric"=-6554654654564.0, "String"="safdsfa", "Boolean"=FALSE}, {"Numeric"=1e+20, "String"="asdfasd", "Boolean"=FALSE}, {"Numeric"=2.0, "String"="afd", "Boolean"=TRUE}, {"Numeric"=12.34, "String"="data", "Boolean"=FALSE}], "string"="strings", "Null array"=[0]} ("Test Config")
        n119 = call "Init OOB.vi"("error in (no error)"=w445) -> ("error out"=w451:errorcluster, "OOB out"=w449:refnum<class "CIFOutOfBand.lvclass">)  [unwired: 9 in]
        n120 = To Variant(anything=w446) -> (Variant=w450:variant)
        n121 = call "Write Local OOB Data.vi"("error in"=w451, "Local OOB Data"=w450, "OOB in"=w449) -> ("error out"=w447:errorcluster, "OOB out"=w448:refnum<class "CIFOutOfBand.lvclass">)  [unwired: 7 in]
        n122 = node-c288() -> (w469:T1)
        n123 = node-c288() -> (w467:T1)
        n124 = timed-loop {
          timing: w469 -> [_]
          timing-out: [_] -> w468
          tunnel: w448 -> [w559]
          tunnel: w447 -> [w558]
          tunnel: [w554] -> w461
          tunnel: [w552] -> w460
          tunnel: [w550] -> w465
          tunnel: [w549] -> w464
          tunnel: [w548] -> w462
          tunnel: w446 -> [w546]
          stop <- TRUE stop-if-true
          n125 = flat-sequence {
            tunnel: w558 -> [w562]
            tunnel: w559 -> [w563]
            tunnel: [w563] -> w556
            tunnel: [w562] -> w555
            tunnel: [w561] -> w549
            tunnel: w546 -> [w560]
            tunnel: [w560] -> w545
            tunnel: w556 -> [w569]
            tunnel: w555 -> [w568]
            tunnel: [w567] -> w553
            tunnel: [w566] -> w551
            tunnel: [w565] -> w547
            tunnel: w545 -> [w564]
            tunnel: [w592] -> w554
            tunnel: w553 -> [w592]
            tunnel: [w591] -> w552
            tunnel: w551 -> [w591]
            tunnel: [w590] -> w550
            tunnel: [w589] -> w548
            tunnel: w547 -> [w589]
            frame #0 {
              n126 = call <vilib>:"High Resolution Relative Seconds.vi"() -> ("relative seconds"=w561:dbl)
            }
            frame #1 {
              w565 = 10000
              n127 = for {
                N: w565 -> [_]
                shift-right: [w575] -> w567
                shift-left: w569 -> [w574]
                shift-right: [w571] -> w566
                shift-left: w568 -> [w572]
                shift-right: [w570] -> _
                shift-left: w564 -> [w573]
                n128 = call "Read OOB DVR.vi"("error in"=w572, "OOB in"=w574) -> ("error out"=w576:errorcluster, "New Commands"=w578:bool, "OOB out"=w577:refnum<class "CIFOutOfBand.lvclass">)  [unwired: 6 in, 1 out]
                n129 = case shown="True" w578 {
                  tunnel: w577 -> [w579 w588]
                  tunnel: w576 -> [w580 w587]
                  tunnel: [w579 w585] -> w575
                  tunnel: w573 -> [_ w583]
                  tunnel: [_ w581] -> w570
                  tunnel: [w580 w582] -> w571
                  frame False {
                  }
                  frame True {
                    n130 = call "Read Local OOB Data.vi"("error in"=w587, "OOB in"=w588) -> ("error out"=w586:errorcluster, "Local OOB Data"=w584:variant, "OOB out"=w585:refnum<class "CIFOutOfBand.lvclass">)  [unwired: 7 in]
                    n131 = Variant To Data(error in=w586, type=w583, Variant=w584) -> (data=w581:T14, error out=w582:errorcluster)
                  }
                }
              }
            }
            frame #2 {
              n132 = call <vilib>:"High Resolution Relative Seconds.vi"() -> ("relative seconds"=w590:dbl)
            }
          }
        }
        n133 = disable-structure shown="Disabled" {
          disable-tunnel: w448 -> [w471 _]
          disable-tunnel: w446 -> [w470 _]
          frame Disabled {
            n134 = while {
              tunnel: w471 -> [w474]
              tunnel: w470 -> [w481]
              i -> [w482]
              stop <- w473 stop-if-true
              n135 = Bundle By Name(cluster=w481, "Numeric"=w482) -> (w475:T14)
              n136 = To Variant(anything=w475) -> (Variant=w477:variant)
              n137 = call "Command to Bitwise Command.vi"("OOB Command"=u8 1) -> ("bit command"=w476:u64)  [unwired: 3 in]
              n138 = call "Write Local OOB Data.vi"("Local OOB Data"=w477, "OOB in"=w474) -> ("error out"=w478:errorcluster, "OOB out"=w479:refnum<class "CIFOutOfBand.lvclass">)  [unwired: 8 in]
              n139 = call "Write OOB DVR.vi"("error in"=w478, "Commands (bitwise)"=w476, "OOB in"=w479) -> ("error out"=w473:errorcluster)  [unwired: 7 in, 1 out]
              n140 = Wait (ms)(milliseconds to wait=u32 3000) -> ()  [unwired: 1 out]
            }
          }
          frame Enabled {
          }
        }
        n141 = timed-loop {
          timing: w467 -> [_]
          timing-out: [_] -> w466
          tunnel: w461 -> [w491]
          tunnel: w460 -> [w490]
          tunnel: [w488] -> w454
          tunnel: [w487] -> w453
          tunnel: w446 -> [w486]
          tunnel: [w483] -> w457
          stop <- TRUE stop-if-true
          n142 = for {
            N: 10000 -> [_]
            shift-right: [w503] -> w488
            shift-left: w491 -> [w505]
            shift-right: [w502] -> w487
            shift-left: w490 -> [w504]
            shift-right: [w496] -> w483
            shift-left: 0.0 -> [w497]
            shift-right: [w495] -> _
            shift-left: w486 -> [w501]
            i -> [w493]
            n143 = flat-sequence {
              tunnel: w504 -> [w516]
              tunnel: w505 -> [w517]
              tunnel: [w517] -> w509
              tunnel: [w516] -> w508
              tunnel: [w515] -> w499
              tunnel: w501 -> [w514]
              tunnel: [w514] -> w507
              tunnel: w509 -> [w523]
              tunnel: w508 -> [w521]
              tunnel: [w520] -> w506
              tunnel: w507 -> [w522]
              tunnel: [w519] -> w494
              tunnel: [w518] -> w492
              tunnel: [w540] -> w503
              tunnel: w506 -> [w540]
              tunnel: [w539] -> w502
              tunnel: [w538] -> w500
              tunnel: [w537] -> w495
              tunnel: w494 -> [w537]
              tunnel: w492 -> [w539]
              frame #0 {
                n144 = call <vilib>:"High Resolution Relative Seconds.vi"() -> ("relative seconds"=w515:dbl)
              }
              frame #1 {
                n145 = call "Read OOB DVR.vi"("error in"=w521, "OOB in"=w523) -> ("error out"=w526:errorcluster, "New Commands"=w524:bool, "OOB out"=w525:refnum<class "CIFOutOfBand.lvclass">)  [unwired: 6 in, 1 out]
                n146 = case shown="True" w524 {
                  tunnel: w525 -> [w527 w536]
                  tunnel: w526 -> [w528 w535]
                  tunnel: [w527 w533] -> w520
                  tunnel: w522 -> [_ w531]
                  tunnel: [_ w529] -> w519
                  tunnel: [w528 w530] -> w518
                  frame False {
                  }
                  frame True {
                    n147 = call "Read Local OOB Data.vi"("error in"=w535, "OOB in"=w536) -> ("error out"=w534:errorcluster, "Local OOB Data"=w532:variant, "OOB out"=w533:refnum<class "CIFOutOfBand.lvclass">)  [unwired: 7 in]
                    n148 = Variant To Data(error in=w534, type=w531, Variant=w532) -> (data=w529:T14, error out=w530:errorcluster)
                  }
                }
              }
              frame #2 {
                n149 = call <vilib>:"High Resolution Relative Seconds.vi"() -> ("relative seconds"=w538:dbl)
              }
            }
            n150 = Subtract(x=w500, y=w499) -> (x-y=w498:dbl)
            n151 = case shown="0" w493 {
              tunnel: w498 -> [_ w513]
              tunnel: w497 -> [w510 w512]
              tunnel: [w510 w511] -> w496
              frame 0 {
              }
              frame 1, Default {
                n152 = Max & Min(x=w513, y=w512) -> (max(x,y)=w511:dbl)  [unwired: 1 out]
              }
            }
          }
        }
        "Max no conflict" <- w457
        n153 = node-c288(w468) -> ()  [unwired: 1 out]
        n154 = node-c288(w466) -> ()  [unwired: 1 out]
        n155 = Subtract(x=w465, y=w464) -> (x-y=w463:dbl)
        n156 = Divide(x=w463, y=w462) -> (x/y=w459:dbl)
        "avg no conflict" <- w459
        n157 = Less?(x=w457, y=9e-07) -> (x < y?=w455:bool)
        n158 = Less?(x=w459, y=5e-07) -> ()  [unwired: 1 out]
        n159 = call "Close OOB.vi"("error in"=w453, "OOB in"=w454) -> ("error out"=w452:errorcluster)  [unwired: 9 in]
      }
      frame 4 {
        w600 = u64 0
        n160 = New Data Value Reference(data value=w600, error in=w602) -> (data value reference=w603:refnum<data-value>, error out=w601:errorcluster)
        n161 = node-c288() -> (w618:T1)
        n162 = node-c288() -> (w616:T1)
        n163 = timed-loop {
          timing: w618 -> [_]
          timing-out: [_] -> w617
          tunnel: w603 -> [w686]
          tunnel: w601 -> [w685]
          tunnel: [w681] -> w610
          tunnel: [w679] -> w609
          tunnel: [w677] -> w614
          tunnel: [w676] -> w613
          tunnel: [w675] -> w611
          tunnel: w600 -> [w673]
          stop <- TRUE stop-if-true
          n164 = flat-sequence {
            tunnel: w685 -> [w689]
            tunnel: w686 -> [w690]
            tunnel: [w690] -> w683
            tunnel: [w689] -> w682
            tunnel: [w688] -> w676
            tunnel: w673 -> [w687]
            tunnel: [w687] -> w672
            tunnel: w683 -> [w696]
            tunnel: w682 -> [w695]
            tunnel: [w694] -> w680
            tunnel: [w693] -> w678
            tunnel: [w692] -> w674
            tunnel: w672 -> [w691]
            tunnel: [w705] -> w681
            tunnel: w680 -> [w705]
            tunnel: [w704] -> w679
            tunnel: w678 -> [w704]
            tunnel: [w703] -> w677
            tunnel: [w702] -> w675
            tunnel: w674 -> [w702]
            frame #0 {
              n165 = call <vilib>:"High Resolution Relative Seconds.vi"() -> ("relative seconds"=w688:dbl)
            }
            frame #1 {
              w692 = 10000
              n166 = for {
                N: w692 -> [_]
                shift-right: [w698] -> w694
                shift-left: w696 -> [w700]
                shift-right: [w697] -> w693
                shift-left: w695 -> [_]
                shift-right: [w699] -> _
                shift-left: w691 -> [_]
                n167 = in-place {
                  in-place-border: [w701] -> w699
                  n168 = in-place-dvr #1(w700) -> (w701:u64)  [unwired: 1 out]
                  n169 = in-place-dvr #1(w701) -> (w698:refnum<data-value>, w697:errorcluster)
                }
              }
            }
            frame #2 {
              n170 = call <vilib>:"High Resolution Relative Seconds.vi"() -> ("relative seconds"=w703:dbl)
            }
          }
        }
        n171 = timed-loop {
          timing: w616 -> [_]
          timing-out: [_] -> w615
          tunnel: w610 -> [w632]
          tunnel: w609 -> [w631]
          tunnel: [w629] -> w599
          tunnel: [w628] -> w598
          tunnel: w600 -> [w627]
          tunnel: [w624] -> w606
          stop <- TRUE stop-if-true
          n172 = for {
            N: 10000 -> [_]
            shift-right: [w644] -> w629
            shift-left: w632 -> [w646]
            shift-right: [w643] -> w628
            shift-left: w631 -> [w645]
            shift-right: [w637] -> w624
            shift-left: 0.0 -> [w638]
            shift-right: [w636] -> _
            shift-left: w627 -> [w642]
            i -> [w634]
            n173 = flat-sequence {
              tunnel: w645 -> [w657]
              tunnel: w646 -> [w658]
              tunnel: [w658] -> w650
              tunnel: [w657] -> w649
              tunnel: [w656] -> w640
              tunnel: w642 -> [w655]
              tunnel: [w655] -> w648
              tunnel: w650 -> [w662]
              tunnel: w649 -> [_]
              tunnel: [w660] -> w647
              tunnel: w648 -> [_]
              tunnel: [w661] -> w635
              tunnel: [w659] -> w633
              tunnel: [w667] -> w644
              tunnel: w647 -> [w667]
              tunnel: [w666] -> w643
              tunnel: [w665] -> w641
              tunnel: [w664] -> w636
              tunnel: w635 -> [w664]
              tunnel: w633 -> [w666]
              frame #0 {
                n174 = call <vilib>:"High Resolution Relative Seconds.vi"() -> ("relative seconds"=w656:dbl)
              }
              frame #1 {
                n175 = in-place {
                  in-place-border: [w663] -> w661
                  n176 = in-place-dvr #2(w662) -> (w663:u64)  [unwired: 1 out]
                  n177 = in-place-dvr #2(w663) -> (w660:refnum<data-value>, w659:errorcluster)
                }
              }
              frame #2 {
                n178 = call <vilib>:"High Resolution Relative Seconds.vi"() -> ("relative seconds"=w665:dbl)
              }
            }
            n179 = Subtract(x=w641, y=w640) -> (x-y=w639:dbl)
            n180 = case shown="0" w634 {
              tunnel: w639 -> [_ w654]
              tunnel: w638 -> [w651 w653]
              tunnel: [w651 w652] -> w637
              frame 0 {
              }
              frame 1, Default {
                n181 = Max & Min(x=w654, y=w653) -> (max(x,y)=w652:dbl)  [unwired: 1 out]
              }
            }
          }
        }
        "Max raw dvr" <- w606
        n182 = while {
          tunnel: w603 -> [w622]
          i -> [w621]
          stop <- w619 stop-if-true
          n183 = To Unsigned Quad Integer(1:w621) -> (0:w620:u64)
          n184 = in-place {
            in-place-border: w620 -> [w623]
            n185 = in-place-dvr #3(w622) -> ()  [unwired: 2 out]
            n186 = in-place-dvr #3(w623) -> (w619:errorcluster)  [unwired: 1 out]
          }
        }
        n187 = node-c288(w617) -> ()  [unwired: 1 out]
        n188 = node-c288(w615) -> ()  [unwired: 1 out]
        n189 = Subtract(x=w614, y=w613) -> (x-y=w612:dbl)
        n190 = Divide(x=w612, y=w611) -> (x/y=w608:dbl)
        "avg raw dvr" <- w608
        n191 = Less?(x=w606, y=9e-07) -> (x < y?=w604:bool)
        n192 = Delete Data Value Reference(data value reference=w599, error in=w598) -> (error out=w597:errorcluster)  [unwired: 1 out]
        n193 = Less?(x=w608, y=5e-07) -> ()  [unwired: 1 out]
      }
      frame 5 {
        w713 = u64 0
        n194 = New Data Value Reference(data value=w713, error in=w715) -> (data value reference=w716:refnum<data-value>, error out=w714:errorcluster)
        n195 = node-c288() -> (w731:T1)
        n196 = node-c288() -> (w729:T1)
        n197 = timed-loop {
          timing: w731 -> [_]
          timing-out: [_] -> w730
          tunnel: w716 -> [w804]
          tunnel: w714 -> [w803]
          tunnel: [w799] -> w723
          tunnel: [w797] -> w722
          tunnel: [w795] -> w727
          tunnel: [w794] -> w726
          tunnel: [w793] -> w724
          tunnel: w713 -> [w791]
          stop <- TRUE stop-if-true
          n198 = flat-sequence {
            tunnel: w803 -> [w807]
            tunnel: w804 -> [w808]
            tunnel: [w808] -> w801
            tunnel: [w807] -> w800
            tunnel: [w806] -> w794
            tunnel: w791 -> [w805]
            tunnel: [w805] -> w790
            tunnel: w801 -> [w814]
            tunnel: w800 -> [w813]
            tunnel: [w812] -> w798
            tunnel: [w811] -> w796
            tunnel: [w810] -> w792
            tunnel: w790 -> [w809]
            tunnel: [w825] -> w799
            tunnel: w798 -> [w825]
            tunnel: [w824] -> w797
            tunnel: w796 -> [w824]
            tunnel: [w823] -> w795
            tunnel: [w822] -> w793
            tunnel: w792 -> [w822]
            frame #0 {
              n199 = call <vilib>:"High Resolution Relative Seconds.vi"() -> ("relative seconds"=w806:dbl)
            }
            frame #1 {
              w810 = 10000
              n200 = for {
                N: w810 -> [_]
                shift-right: [w818] -> w812
                shift-left: w814 -> [w820]
                shift-right: [w817] -> w811
                shift-left: w813 -> [_]
                shift-right: [w819] -> _
                shift-left: w809 -> [_]
                i -> [w816]
                n201 = To Unsigned Quad Integer(1:w816) -> (0:w815:u64)
                n202 = in-place {
                  in-place-border: [w821] -> w819
                  in-place-border: w815 -> [w821]
                  n203 = in-place-dvr #4(w820) -> ()  [unwired: 2 out]
                  n204 = in-place-dvr #4(w821) -> (w818:refnum<data-value>, w817:errorcluster)
                }
              }
            }
            frame #2 {
              n205 = call <vilib>:"High Resolution Relative Seconds.vi"() -> ("relative seconds"=w823:dbl)
            }
          }
        }
        n206 = timed-loop {
          timing: w729 -> [_]
          timing-out: [_] -> w728
          tunnel: w723 -> [w746]
          tunnel: w722 -> [w745]
          tunnel: [w743] -> w712
          tunnel: [w742] -> w711
          tunnel: w713 -> [w741]
          tunnel: [w738] -> w719
          stop <- TRUE stop-if-true
          n207 = for {
            N: 10000 -> [_]
            shift-right: [w760] -> w743
            shift-left: w746 -> [w762]
            shift-right: [w759] -> w742
            shift-left: w745 -> [w761]
            shift-right: [w753] -> w738
            shift-left: 0.0 -> [w754]
            shift-right: [w752] -> _
            shift-left: w741 -> [w758]
            i -> [w749]
            n208 = To Unsigned Quad Integer(1:w749) -> (0:w748:u64)
            n209 = flat-sequence {
              tunnel: w761 -> [w774]
              tunnel: w762 -> [w775]
              tunnel: [w775] -> w766
              tunnel: [w774] -> w765
              tunnel: [w773] -> w756
              tunnel: w758 -> [w772]
              tunnel: [w772] -> w764
              tunnel: w748 -> [w771]
              tunnel: [w771] -> w747
              tunnel: w766 -> [w780]
              tunnel: w765 -> [_]
              tunnel: [w778] -> w763
              tunnel: w764 -> [_]
              tunnel: [w779] -> w751
              tunnel: [w777] -> w750
              tunnel: w747 -> [w776]
              tunnel: [w785] -> w760
              tunnel: w763 -> [w785]
              tunnel: [w784] -> w759
              tunnel: [w783] -> w757
              tunnel: [w782] -> w752
              tunnel: w751 -> [w782]
              tunnel: w750 -> [w784]
              frame #0 {
                n210 = call <vilib>:"High Resolution Relative Seconds.vi"() -> ("relative seconds"=w773:dbl)
              }
              frame #1 {
                n211 = in-place {
                  in-place-border: [w781] -> w779
                  in-place-border: w776 -> [w781]
                  n212 = in-place-dvr #5(w780) -> ()  [unwired: 2 out]
                  n213 = in-place-dvr #5(w781) -> (w778:refnum<data-value>, w777:errorcluster)
                }
              }
              frame #2 {
                n214 = call <vilib>:"High Resolution Relative Seconds.vi"() -> ("relative seconds"=w783:dbl)
              }
            }
            n215 = Subtract(x=w757, y=w756) -> (x-y=w755:dbl)
            n216 = case shown="0" w749 {
              tunnel: w755 -> [_ w770]
              tunnel: w754 -> [w767 w769]
              tunnel: [w767 w768] -> w753
              frame 0 {
              }
              frame 1, Default {
                n217 = Max & Min(x=w770, y=w769) -> (max(x,y)=w768:dbl)  [unwired: 1 out]
              }
            }
          }
        }
        "Max raw dvr write" <- w719
        n218 = while {
          tunnel: w716 -> [w736]
          tunnel: [w732] -> _
          i -> [w735]
          stop <- w733 stop-if-true
          n219 = To Unsigned Quad Integer(1:w735) -> (0:w734:u64)
          n220 = in-place {
            in-place-border: w734 -> [_]
            in-place-border: [w737] -> w732
            n221 = in-place-dvr #6(w736) -> (w737:u64)  [unwired: 1 out]
            n222 = in-place-dvr #6(w737) -> (w733:errorcluster)  [unwired: 1 out]
          }
        }
        n223 = node-c288(w730) -> ()  [unwired: 1 out]
        n224 = node-c288(w728) -> ()  [unwired: 1 out]
        n225 = Subtract(x=w727, y=w726) -> (x-y=w725:dbl)
        n226 = Divide(x=w725, y=w724) -> (x/y=w721:dbl)
        "avg raw dvr write" <- w721
        n227 = Less?(x=w719, y=9e-07) -> (x < y?=w717:bool)
        n228 = Delete Data Value Reference(data value reference=w712, error in=w711) -> (error out=w710:errorcluster)  [unwired: 1 out]
        n229 = Less?(x=w721, y=5e-07) -> ()  [unwired: 1 out]
      }
      frame 0 {
        w835 = u64 0
        n230 = RT FIFO Create(1:w835, 3:w833, 4:u32 1 ("size (10)"), 7:T4 {"read mode"=enum."polling", "write mode"=enum."polling"} ("r/w modes (polling,polling)")) -> (8:w834:refnum<k33>, 11:w832:errorcluster)  [unwired: 4 in, 1 out]
        n231 = node-c288() -> (w853:T1)
        n232 = node-c288() -> (w851:T1)
        n233 = timed-loop {
          timing: w853 -> [_]
          timing-out: [_] -> w852
          tunnel: w834 -> [w924]
          tunnel: w832 -> [w923]
          tunnel: [w919] -> w845
          tunnel: [w917] -> w844
          tunnel: [w915] -> w849
          tunnel: [w914] -> w848
          tunnel: [w913] -> w846
          tunnel: w835 -> [w911]
          stop <- TRUE stop-if-true
          n234 = flat-sequence {
            tunnel: w923 -> [w927]
            tunnel: w924 -> [w928]
            tunnel: [w928] -> w921
            tunnel: [w927] -> w920
            tunnel: [w926] -> w914
            tunnel: w911 -> [w925]
            tunnel: [w925] -> w910
            tunnel: w921 -> [w934]
            tunnel: w920 -> [w933]
            tunnel: [w932] -> w918
            tunnel: [w931] -> w916
            tunnel: [w930] -> w912
            tunnel: w910 -> [w929]
            tunnel: [w945] -> w919
            tunnel: w918 -> [w945]
            tunnel: [w944] -> w917
            tunnel: w916 -> [w944]
            tunnel: [w943] -> w915
            tunnel: [w942] -> w913
            tunnel: w912 -> [w942]
            frame #0 {
              n235 = call <vilib>:"High Resolution Relative Seconds.vi"() -> ("relative seconds"=w926:dbl)
            }
            frame #1 {
              w930 = 10000
              n236 = for {
                N: w930 -> [_]
                shift-right: [w939] -> w932
                shift-left: w934 -> [w940]
                shift-right: [w935] -> w931
                shift-left: w933 -> [w938]
                shift-right: [w936] -> _
                shift-left: w929 -> [w937]
                i -> [w941]
                n237 = To Unsigned Quad Integer(1:w941) -> ()  [unwired: 1 out]
                n238 = RT FIFO Read(0:w940, 1:w937, 3:w938) -> (8:w939:refnum<k33>, 9:w936:u64, 11:w935:errorcluster)  [unwired: 1 in, 2 out]
              }
            }
            frame #2 {
              n239 = call <vilib>:"High Resolution Relative Seconds.vi"() -> ("relative seconds"=w943:dbl)
            }
          }
        }
        n240 = timed-loop {
          timing: w851 -> [_]
          timing-out: [_] -> w850
          tunnel: w845 -> [w866]
          tunnel: w844 -> [w865]
          tunnel: [w863] -> w838
          tunnel: [w862] -> w837
          tunnel: w835 -> [w861]
          tunnel: [w858] -> w841
          stop <- TRUE stop-if-true
          n241 = for {
            N: 10000 -> [_]
            shift-right: [w880] -> w863
            shift-left: w866 -> [w882]
            shift-right: [w879] -> w862
            shift-left: w865 -> [w881]
            shift-right: [w873] -> w858
            shift-left: 0.0 -> [w874]
            shift-right: [w872] -> _
            shift-left: w861 -> [w878]
            i -> [w869]
            n242 = To Unsigned Quad Integer(1:w869) -> (0:w868:u64)
            n243 = flat-sequence {
              tunnel: w881 -> [w894]
              tunnel: w882 -> [w895]
              tunnel: [w895] -> w886
              tunnel: [w894] -> w885
              tunnel: [w893] -> w876
              tunnel: w878 -> [w892]
              tunnel: [w892] -> w884
              tunnel: w868 -> [w891]
              tunnel: [w891] -> w867
              tunnel: w886 -> [w901]
              tunnel: w885 -> [w899]
              tunnel: [w900] -> w883
              tunnel: w884 -> [w898]
              tunnel: [w897] -> w871
              tunnel: [w896] -> w870
              tunnel: w867 -> [_]
              tunnel: [w905] -> w880
              tunnel: w883 -> [w905]
              tunnel: [w904] -> w879
              tunnel: [w903] -> w877
              tunnel: [w902] -> w872
              tunnel: w871 -> [w902]
              tunnel: w870 -> [w904]
              frame #0 {
                n244 = call <vilib>:"High Resolution Relative Seconds.vi"() -> ("relative seconds"=w893:dbl)
              }
              frame #1 {
                n245 = RT FIFO Read(0:w901, 1:w898, 3:w899) -> (8:w900:refnum<k33>, 9:w897:u64, 11:w896:errorcluster)  [unwired: 1 in, 2 out]
              }
              frame #2 {
                n246 = call <vilib>:"High Resolution Relative Seconds.vi"() -> ("relative seconds"=w903:dbl)
              }
            }
            n247 = Subtract(x=w877, y=w876) -> (x-y=w875:dbl)
            n248 = case shown="0" w869 {
              tunnel: w875 -> [_ w890]
              tunnel: w874 -> [w887 w889]
              tunnel: [w887 w888] -> w873
              frame 0 {
              }
              frame 1, Default {
                n249 = Max & Min(x=w890, y=w889) -> (max(x,y)=w888:dbl)  [unwired: 1 out]
              }
            }
          }
        }
        "Max RTFifo" <- w841
        n250 = while {
          tunnel: w834 -> [w856]
          i -> [w857]
          stop <- w854 stop-if-true
          n251 = To Unsigned Quad Integer(1:w857) -> (0:w855:u64)
          n252 = RT FIFO Write(0:w856, 1:w855) -> (11:w854:errorcluster)  [unwired: 3 in, 3 out]
        }
        n253 = node-c288(w852) -> ()  [unwired: 1 out]
        n254 = node-c288(w850) -> ()  [unwired: 1 out]
        n255 = Subtract(x=w849, y=w848) -> (x-y=w847:dbl)
        n256 = Divide(x=w847, y=w846) -> (x/y=w843:dbl)
        "avg RTFifo" <- w843
        n257 = Less?(x=w841, y=9e-07) -> (x < y?=w839:bool)
        n258 = RT FIFO Delete(0:w838, 3:w837) -> (11:w836:errorcluster)  [unwired: 1 in]
        n259 = Less?(x=w843, y=5e-07) -> ()  [unwired: 1 out]
      }
      frame 7 {
        w953 = u64 0
        n260 = Obtain Notifier(notification data type=w953, error in (no error)=w951) -> (notifier out=w952:refnum<notifier>, error out=w950:errorcluster)  [unwired: 2 in, 1 out]
        n261 = node-c288() -> (w971:T1)
        n262 = node-c288() -> (w969:T1)
        n263 = timed-loop {
          timing: w971 -> [_]
          timing-out: [_] -> w970
          tunnel: w952 -> [w1042]
          tunnel: w950 -> [w1041]
          tunnel: [w1037] -> w963
          tunnel: [w1035] -> w962
          tunnel: [w1033] -> w967
          tunnel: [w1032] -> w966
          tunnel: [w1031] -> w964
          tunnel: w953 -> [w1029]
          stop <- TRUE stop-if-true
          n264 = flat-sequence {
            tunnel: w1041 -> [w1045]
            tunnel: w1042 -> [w1046]
            tunnel: [w1046] -> w1039
            tunnel: [w1045] -> w1038
            tunnel: [w1044] -> w1032
            tunnel: w1029 -> [w1043]
            tunnel: [w1043] -> w1028
            tunnel: w1039 -> [w1052]
            tunnel: w1038 -> [w1051]
            tunnel: [w1050] -> w1036
            tunnel: [w1049] -> w1034
            tunnel: [w1048] -> w1030
            tunnel: w1028 -> [w1047]
            tunnel: [w1063] -> w1037
            tunnel: w1036 -> [w1063]
            tunnel: [w1062] -> w1035
            tunnel: w1034 -> [w1062]
            tunnel: [w1061] -> w1033
            tunnel: [w1060] -> w1031
            tunnel: w1030 -> [w1060]
            frame #0 {
              n265 = call <vilib>:"High Resolution Relative Seconds.vi"() -> ("relative seconds"=w1044:dbl)
            }
            frame #1 {
              w1048 = 10000
              n266 = for {
                N: w1048 -> [_]
                shift-right: [w1057] -> w1050
                shift-left: w1052 -> [w1058]
                shift-right: [w1054] -> w1049
                shift-left: w1051 -> [w1056]
                shift-right: [w1055] -> _
                shift-left: w1047 -> [_]
                i -> [w1059]
                n267 = To Unsigned Quad Integer(1:w1059) -> ()  [unwired: 1 out]
                n268 = Wait on Notification(notifier=w1058, timeout in ms (-1)=0, error in (no error)=w1056) -> (notifier out=w1057:refnum<notifier>, notification=w1055:u64, error out=w1054:errorcluster)  [unwired: 1 in, 1 out]
              }
            }
            frame #2 {
              n269 = call <vilib>:"High Resolution Relative Seconds.vi"() -> ("relative seconds"=w1061:dbl)
            }
          }
        }
        n270 = timed-loop {
          timing: w969 -> [_]
          timing-out: [_] -> w968
          tunnel: w963 -> [w984]
          tunnel: w962 -> [w983]
          tunnel: [w981] -> w956
          tunnel: [w980] -> w955
          tunnel: w953 -> [w979]
          tunnel: [w976] -> w959
          stop <- TRUE stop-if-true
          n271 = for {
            N: 10000 -> [_]
            shift-right: [w998] -> w981
            shift-left: w984 -> [w1000]
            shift-right: [w997] -> w980
            shift-left: w983 -> [w999]
            shift-right: [w991] -> w976
            shift-left: 0.0 -> [w992]
            shift-right: [w990] -> _
            shift-left: w979 -> [w996]
            i -> [w987]
            n272 = To Unsigned Quad Integer(1:w987) -> (0:w986:u64)
            n273 = flat-sequence {
              tunnel: w999 -> [w1012]
              tunnel: w1000 -> [w1013]
              tunnel: [w1013] -> w1004
              tunnel: [w1012] -> w1003
              tunnel: [w1011] -> w994
              tunnel: w996 -> [w1010]
              tunnel: [w1010] -> w1002
              tunnel: w986 -> [w1009]
              tunnel: [w1009] -> w985
              tunnel: w1004 -> [w1019]
              tunnel: w1003 -> [w1017]
              tunnel: [w1018] -> w1001
              tunnel: w1002 -> [_]
              tunnel: [w1016] -> w989
              tunnel: [w1015] -> w988
              tunnel: w985 -> [_]
              tunnel: [w1023] -> w998
              tunnel: w1001 -> [w1023]
              tunnel: [w1022] -> w997
              tunnel: [w1021] -> w995
              tunnel: [w1020] -> w990
              tunnel: w989 -> [w1020]
              tunnel: w988 -> [w1022]
              frame #0 {
                n274 = call <vilib>:"High Resolution Relative Seconds.vi"() -> ("relative seconds"=w1011:dbl)
              }
              frame #1 {
                n275 = Wait on Notification(notifier=w1019, timeout in ms (-1)=0, error in (no error)=w1017) -> (notifier out=w1018:refnum<notifier>, notification=w1016:u64, error out=w1015:errorcluster)  [unwired: 1 in, 1 out]
              }
              frame #2 {
                n276 = call <vilib>:"High Resolution Relative Seconds.vi"() -> ("relative seconds"=w1021:dbl)
              }
            }
            n277 = Subtract(x=w995, y=w994) -> (x-y=w993:dbl)
            n278 = case shown="0" w987 {
              tunnel: w993 -> [_ w1008]
              tunnel: w992 -> [w1005 w1007]
              tunnel: [w1005 w1006] -> w991
              frame 0 {
              }
              frame 1, Default {
                n279 = Max & Min(x=w1008, y=w1007) -> (max(x,y)=w1006:dbl)  [unwired: 1 out]
              }
            }
          }
        }
        "Max Notifier" <- w959
        n280 = while {
          tunnel: w952 -> [w974]
          i -> [w975]
          stop <- w972 stop-if-true
          n281 = To Unsigned Quad Integer(1:w975) -> (0:w973:u64)
          n282 = Send Notification(notification=w973, notifier=w974) -> (error out=w972:errorcluster)  [unwired: 1 in, 1 out]
        }
        n283 = node-c288(w970) -> ()  [unwired: 1 out]
        n284 = node-c288(w968) -> ()  [unwired: 1 out]
        n285 = Subtract(x=w967, y=w966) -> (x-y=w965:dbl)
        n286 = Divide(x=w965, y=w964) -> (x/y=w961:dbl)
        "avg Notifier" <- w961
        n287 = Less?(x=w959, y=9e-07) -> (x < y?=w957:bool)
        n288 = Release Notifier(notifier=w956, error in (no error)=w955) -> (error out=w954:errorcluster)  [unwired: 1 in, 2 out]
        n289 = Less?(x=w961, y=5e-07) -> ()  [unwired: 1 out]
      }
      frame 8 {
        w1073 = u64 0
        n290 = Generate Occurrence() -> (w1072:refnum<k4>)
        n291 = flat-sequence {
          tunnel: [w1092] -> w1069
          frame #0 {
            w1092 = FALSE ("stop")
            n292 = local write "stop"(w1092) -> ()
          }
        }
        n293 = node-c288() -> (w1088:T1)
        n294 = node-c288() -> (w1086:T1)
        n295 = timed-loop {
          timing: w1088 -> [_]
          timing-out: [_] -> w1087
          tunnel: w1072 -> [w1158]
          tunnel: w1071 -> [w1157]
          tunnel: [w1153] -> w1080
          tunnel: [w1151] -> w1079
          tunnel: [w1149] -> w1084
          tunnel: [w1148] -> w1083
          tunnel: [w1147] -> w1081
          tunnel: w1073 -> [w1145]
          stop <- TRUE stop-if-true
          n296 = flat-sequence {
            tunnel: w1157 -> [w1161]
            tunnel: w1158 -> [w1162]
            tunnel: [w1162] -> w1155
            tunnel: [w1161] -> w1154
            tunnel: [w1160] -> w1148
            tunnel: w1145 -> [w1159]
            tunnel: [w1159] -> w1144
            tunnel: w1155 -> [w1168]
            tunnel: w1154 -> [w1167]
            tunnel: [w1166] -> w1152
            tunnel: [w1165] -> w1150
            tunnel: [w1164] -> w1146
            tunnel: w1144 -> [w1163]
            tunnel: [w1177] -> w1153
            tunnel: w1152 -> [w1177]
            tunnel: [w1176] -> w1151
            tunnel: w1150 -> [w1176]
            tunnel: [w1175] -> w1149
            tunnel: [w1174] -> w1147
            tunnel: w1146 -> [w1174]
            frame #0 {
              n297 = call <vilib>:"High Resolution Relative Seconds.vi"() -> ("relative seconds"=w1160:dbl)
            }
            frame #1 {
              w1164 = 10000
              n298 = for {
                N: w1164 -> [_]
                shift-right: [w1170] -> w1166
                shift-left: w1168 -> [w1170]
                shift-right: [w1171] -> w1165
                shift-left: w1167 -> [w1171]
                shift-right: [w1169] -> _
                shift-left: w1163 -> [w1169]
                i -> [w1173]
                n299 = To Unsigned Quad Integer(1:w1173) -> ()  [unwired: 1 out]
                n300 = Wait on Occurrence(2:w1170, 3:0 ("timeout in ms (-1)")) -> ()  [unwired: 1 in, 1 out]
              }
            }
            frame #2 {
              n301 = call <vilib>:"High Resolution Relative Seconds.vi"() -> ("relative seconds"=w1175:dbl)
            }
          }
        }
        n302 = timed-loop {
          timing: w1086 -> [_]
          timing-out: [_] -> w1085
          tunnel: w1080 -> [w1102]
          tunnel: w1079 -> [w1101]
          tunnel: [w1099] -> _
          tunnel: [w1098] -> w1070
          tunnel: w1073 -> [w1097]
          tunnel: [w1094] -> w1076
          tunnel: [TRUE] -> w1068
          stop <- TRUE stop-if-true
          n303 = for {
            N: 10000 -> [_]
            shift-right: [w1116] -> w1099
            shift-left: w1102 -> [w1118]
            shift-right: [w1115] -> w1098
            shift-left: w1101 -> [w1117]
            shift-right: [w1109] -> w1094
            shift-left: 0.0 -> [w1110]
            shift-right: [w1108] -> _
            shift-left: w1097 -> [w1114]
            i -> [w1105]
            n304 = To Unsigned Quad Integer(1:w1105) -> (0:w1104:u64)
            n305 = flat-sequence {
              tunnel: w1117 -> [w1130]
              tunnel: w1118 -> [w1131]
              tunnel: [w1131] -> w1122
              tunnel: [w1130] -> w1121
              tunnel: [w1129] -> w1112
              tunnel: w1114 -> [w1128]
              tunnel: [w1128] -> w1120
              tunnel: w1104 -> [w1127]
              tunnel: [w1127] -> w1103
              tunnel: w1122 -> [w1135]
              tunnel: w1121 -> [w1133]
              tunnel: [w1135] -> w1119
              tunnel: w1120 -> [w1132]
              tunnel: [w1132] -> w1107
              tunnel: [w1133] -> w1106
              tunnel: w1103 -> [_]
              tunnel: [w1139] -> w1116
              tunnel: w1119 -> [w1139]
              tunnel: [w1138] -> w1115
              tunnel: [w1137] -> w1113
              tunnel: [w1136] -> w1108
              tunnel: w1107 -> [w1136]
              tunnel: w1106 -> [w1138]
              frame #0 {
                n306 = call <vilib>:"High Resolution Relative Seconds.vi"() -> ("relative seconds"=w1129:dbl)
              }
              frame #1 {
                n307 = Wait on Occurrence(2:w1135, 3:0 ("timeout in ms (-1)")) -> ()  [unwired: 1 in, 1 out]
              }
              frame #2 {
                n308 = call <vilib>:"High Resolution Relative Seconds.vi"() -> ("relative seconds"=w1137:dbl)
              }
            }
            n309 = Subtract(x=w1113, y=w1112) -> (x-y=w1111:dbl)
            n310 = case shown="0" w1105 {
              tunnel: w1111 -> [_ w1126]
              tunnel: w1110 -> [w1123 w1125]
              tunnel: [w1123 w1124] -> w1109
              frame 0 {
              }
              frame 1, Default {
                n311 = Max & Min(x=w1126, y=w1125) -> (max(x,y)=w1124:dbl)  [unwired: 1 out]
              }
            }
          }
        }
        "Max Occur" <- w1076
        n312 = while {
          tunnel: w1072 -> [w1090]
          tunnel: w1069 -> [_]
          i -> [w1091]
          stop <- w1089 stop-if-true
          n313 = To Unsigned Quad Integer(1:w1091) -> ()  [unwired: 1 out]
          n314 = Set Occurrence(w1090) -> ()
          n315 = local read "stop"() -> (w1089:bool)
        }
        n316 = node-c288(w1087) -> ()  [unwired: 1 out]
        n317 = node-c288(w1085) -> ()  [unwired: 1 out]
        n318 = local write "stop"(w1068) -> ()
        n319 = Subtract(x=w1084, y=w1083) -> (x-y=w1082:dbl)
        n320 = Divide(x=w1082, y=w1081) -> (x/y=w1078:dbl)
        "avg Occur" <- w1078
        n321 = Less?(x=w1076, y=9e-07) -> (x < y?=w1074:bool)
        n322 = Less?(x=w1078, y=5e-07) -> ()  [unwired: 1 out]
      }
      frame 9 {
        w1188 = T14 {"Numeric"=54.0, "Array"=[{"Numeric"=3.1415, "String"="strings are fun especially when they are pretty long. a;lfkjasd;lkfjsd;lkfjsd;lkfj;dslkfj ;dslkjf f;ldskjff ;dskfj;s dlkfj;dslk jfj;dslkk jfs\ndsajf'sdjkf ;dsaf\nsjd f'\nsdafkjj'lds kf sda\nf jdsa'", "Boolean"=FALSE}, {"Numeric"=-6554654654564.0, "String"="safdsfa", "Boolean"=FALSE}, {"Numeric"=1e+20, "String"="asdfasd", "Boolean"=FALSE}, {"Numeric"=2.0, "String"="afd", "Boolean"=TRUE}, {"Numeric"=12.34, "String"="data", "Boolean"=FALSE}], "string"="strings", "Null array"=[0]} ("Test Config")
        n323 = Obtain Notifier(notification data type=w1188, error in (no error)=w1187) -> (notifier out=w1185:refnum<notifier>, error out=w1186:errorcluster)  [unwired: 2 in, 1 out]
        n324 = node-c288() -> (w1203:T1)
        n325 = node-c288() -> (w1201:T1)
        n326 = timed-loop {
          timing: w1203 -> [_]
          timing-out: [_] -> w1202
          tunnel: w1185 -> [w1272]
          tunnel: w1186 -> [w1271]
          tunnel: [w1267] -> w1195
          tunnel: [w1265] -> w1194
          tunnel: [w1263] -> w1199
          tunnel: [w1262] -> w1198
          tunnel: [w1261] -> w1196
          tunnel: w1188 -> [w1259]
          stop <- TRUE stop-if-true
          n327 = flat-sequence {
            tunnel: w1271 -> [w1275]
            tunnel: w1272 -> [w1276]
            tunnel: [w1276] -> w1269
            tunnel: [w1275] -> w1268
            tunnel: [w1274] -> w1262
            tunnel: w1259 -> [w1273]
            tunnel: [w1273] -> w1258
            tunnel: w1269 -> [w1282]
            tunnel: w1268 -> [w1281]
            tunnel: [w1280] -> w1266
            tunnel: [w1279] -> w1264
            tunnel: [w1278] -> w1260
            tunnel: w1258 -> [w1277]
            tunnel: [w1292] -> w1267
            tunnel: w1266 -> [w1292]
            tunnel: [w1291] -> w1265
            tunnel: w1264 -> [w1291]
            tunnel: [w1290] -> w1263
            tunnel: [w1289] -> w1261
            tunnel: w1260 -> [w1289]
            frame #0 {
              n328 = call <vilib>:"High Resolution Relative Seconds.vi"() -> ("relative seconds"=w1274:dbl)
            }
            frame #1 {
              w1278 = 10000
              n329 = for {
                N: w1278 -> [_]
                shift-right: [w1287] -> w1280
                shift-left: w1282 -> [w1288]
                shift-right: [w1286] -> w1279
                shift-left: w1281 -> [w1285]
                shift-right: [w1284] -> _
                shift-left: w1277 -> [_]
                n330 = Wait on Notification(notifier=w1288, timeout in ms (-1)=0, error in (no error)=w1285) -> (notifier out=w1287:refnum<notifier>, notification=w1284:T14, error out=w1286:errorcluster)  [unwired: 1 in, 1 out]
              }
            }
            frame #2 {
              n331 = call <vilib>:"High Resolution Relative Seconds.vi"() -> ("relative seconds"=w1290:dbl)
            }
          }
        }
        n332 = timed-loop {
          timing: w1201 -> [_]
          timing-out: [_] -> w1200
          tunnel: w1195 -> [w1217]
          tunnel: w1194 -> [w1216]
          tunnel: [w1214] -> w1184
          tunnel: [w1213] -> w1183
          tunnel: w1188 -> [w1212]
          tunnel: [w1209] -> w1191
          stop <- TRUE stop-if-true
          n333 = for {
            N: 10000 -> [_]
            shift-right: [w1229] -> w1214
            shift-left: w1217 -> [w1231]
            shift-right: [w1228] -> w1213
            shift-left: w1216 -> [w1230]
            shift-right: [w1222] -> w1209
            shift-left: 0.0 -> [w1223]
            shift-right: [w1221] -> _
            shift-left: w1212 -> [w1227]
            i -> [w1219]
            n334 = flat-sequence {
              tunnel: w1230 -> [w1242]
              tunnel: w1231 -> [w1243]
              tunnel: [w1243] -> w1235
              tunnel: [w1242] -> w1234
              tunnel: [w1241] -> w1225
              tunnel: w1227 -> [w1240]
              tunnel: [w1240] -> w1233
              tunnel: w1235 -> [w1249]
              tunnel: w1234 -> [w1246]
              tunnel: [w1248] -> w1232
              tunnel: w1233 -> [_]
              tunnel: [w1245] -> w1220
              tunnel: [w1247] -> w1218
              tunnel: [w1253] -> w1229
              tunnel: w1232 -> [w1253]
              tunnel: [w1252] -> w1228
              tunnel: [w1251] -> w1226
              tunnel: [w1250] -> w1221
              tunnel: w1220 -> [w1250]
              tunnel: w1218 -> [w1252]
              frame #0 {
                n335 = call <vilib>:"High Resolution Relative Seconds.vi"() -> ("relative seconds"=w1241:dbl)
              }
              frame #1 {
                n336 = Wait on Notification(notifier=w1249, timeout in ms (-1)=0, error in (no error)=w1246) -> (notifier out=w1248:refnum<notifier>, notification=w1245:T14, error out=w1247:errorcluster)  [unwired: 1 in, 1 out]
              }
              frame #2 {
                n337 = call <vilib>:"High Resolution Relative Seconds.vi"() -> ("relative seconds"=w1251:dbl)
              }
            }
            n338 = Subtract(x=w1226, y=w1225) -> (x-y=w1224:dbl)
            n339 = case shown="0" w1219 {
              tunnel: w1224 -> [_ w1239]
              tunnel: w1223 -> [w1236 w1238]
              tunnel: [w1236 w1237] -> w1222
              frame 0 {
              }
              frame 1, Default {
                n340 = Max & Min(x=w1239, y=w1238) -> (max(x,y)=w1237:dbl)  [unwired: 1 out]
              }
            }
          }
        }
        "Max Complexnote" <- w1191
        n341 = while {
          tunnel: w1185 -> [w1206]
          tunnel: w1188 -> [w1207]
          i -> [w1208]
          stop <- w1204 stop-if-true
          n342 = Bundle By Name(cluster=w1207, "Numeric"=w1208) -> (w1205:T14)
          n343 = Send Notification(notification=w1205, notifier=w1206) -> (error out=w1204:errorcluster)  [unwired: 1 in, 1 out]
        }
        n344 = node-c288(w1202) -> ()  [unwired: 1 out]
        n345 = node-c288(w1200) -> ()  [unwired: 1 out]
        n346 = Subtract(x=w1199, y=w1198) -> (x-y=w1197:dbl)
        n347 = Divide(x=w1197, y=w1196) -> (x/y=w1193:dbl)
        "avg complexnote" <- w1193
        n348 = Less?(x=w1191, y=4e-05) -> (x < y?=w1189:bool)
        n349 = Less?(x=w1193, y=5e-07) -> ()  [unwired: 1 out]
        n350 = Release Notifier(notifier=w1184, error in (no error)=w1183) -> (error out=w1182:errorcluster)  [unwired: 1 in, 2 out]
      }
      frame 10 {
        w1303 = T14 {"Numeric"=54.0, "Array"=[{"Numeric"=3.1415, "String"="strings are fun especially when they are pretty long. a;lfkjasd;lkfjsd;lkfjsd;lkfj;dslkfj ;dslkjf f;ldskjff ;dskfj;s dlkfj;dslk jfj;dslkk jfs\ndsajf'sdjkf ;dsaf\nsjd f'\nsdafkjj'lds kf sda\nf jdsa'", "Boolean"=FALSE}, {"Numeric"=-6554654654564.0, "String"="safdsfa", "Boolean"=FALSE}, {"Numeric"=1e+20, "String"="asdfasd", "Boolean"=FALSE}, {"Numeric"=2.0, "String"="afd", "Boolean"=TRUE}, {"Numeric"=12.34, "String"="data", "Boolean"=FALSE}], "string"="strings", "Null array"=[0]} ("Test Config")
        n351 = Obtain Notifier(notification data type=w1303, error in (no error)=w1302) -> (notifier out=w1300:refnum<notifier>, error out=w1301:errorcluster)  [unwired: 2 in, 1 out]
        n352 = node-c288() -> (w1318:T1)
        n353 = node-c288() -> (w1316:T1)
        n354 = timed-loop {
          timing: w1318 -> [_]
          timing-out: [_] -> w1317
          tunnel: w1300 -> [w1387]
          tunnel: w1301 -> [w1386]
          tunnel: [w1382] -> w1310
          tunnel: [w1380] -> w1309
          tunnel: [w1378] -> w1314
          tunnel: [w1377] -> w1313
          tunnel: [w1376] -> w1311
          tunnel: w1303 -> [w1374]
          stop <- TRUE stop-if-true
          n355 = flat-sequence {
            tunnel: w1386 -> [w1390]
            tunnel: w1387 -> [w1391]
            tunnel: [w1391] -> w1384
            tunnel: [w1390] -> w1383
            tunnel: [w1389] -> w1377
            tunnel: w1374 -> [w1388]
            tunnel: [w1388] -> w1373
            tunnel: w1384 -> [w1397]
            tunnel: w1383 -> [w1396]
            tunnel: [w1395] -> w1381
            tunnel: [w1394] -> w1379
            tunnel: [w1393] -> w1375
            tunnel: w1373 -> [w1392]
            tunnel: [w1406] -> w1382
            tunnel: w1381 -> [w1406]
            tunnel: [w1405] -> w1380
            tunnel: w1379 -> [w1405]
            tunnel: [w1404] -> w1378
            tunnel: [w1403] -> w1376
            tunnel: w1375 -> [w1403]
            frame #0 {
              n356 = call <vilib>:"High Resolution Relative Seconds.vi"() -> ("relative seconds"=w1389:dbl)
            }
            frame #1 {
              w1393 = 10000
              n357 = for {
                N: w1393 -> [_]
                shift-right: [w1399] -> w1395
                shift-left: w1397 -> [w1402]
                shift-right: [w1400] -> w1394
                shift-left: w1396 -> [w1401]
                shift-right: [w1398] -> _
                shift-left: w1392 -> [w1398]
                n358 = Send Notification(notification=w1398, notifier=w1402, error in (no error)=w1401) -> (notifier out=w1399:refnum<notifier>, error out=w1400:errorcluster)
              }
            }
            frame #2 {
              n359 = call <vilib>:"High Resolution Relative Seconds.vi"() -> ("relative seconds"=w1404:dbl)
            }
          }
        }
        n360 = timed-loop {
          timing: w1316 -> [_]
          timing-out: [_] -> w1315
          tunnel: w1310 -> [w1333]
          tunnel: w1309 -> [w1332]
          tunnel: [w1330] -> w1299
          tunnel: [w1329] -> w1298
          tunnel: w1303 -> [w1328]
          tunnel: [w1325] -> w1306
          stop <- TRUE stop-if-true
          n361 = for {
            N: 10000 -> [_]
            shift-right: [w1345] -> w1330
            shift-left: w1333 -> [w1347]
            shift-right: [w1344] -> w1329
            shift-left: w1332 -> [w1346]
            shift-right: [w1338] -> w1325
            shift-left: 0.0 -> [w1339]
            shift-right: [w1337] -> _
            shift-left: w1328 -> [w1343]
            i -> [w1335]
            n362 = flat-sequence {
              tunnel: w1346 -> [w1358]
              tunnel: w1347 -> [w1359]
              tunnel: [w1359] -> w1351
              tunnel: [w1358] -> w1350
              tunnel: [w1357] -> w1341
              tunnel: w1343 -> [w1356]
              tunnel: [w1356] -> w1349
              tunnel: w1351 -> [w1364]
              tunnel: w1350 -> [w1363]
              tunnel: [w1361] -> w1348
              tunnel: w1349 -> [w1360]
              tunnel: [w1360] -> w1336
              tunnel: [w1362] -> w1334
              tunnel: [w1368] -> w1345
              tunnel: w1348 -> [w1368]
              tunnel: [w1367] -> w1344
              tunnel: [w1366] -> w1342
              tunnel: [w1365] -> w1337
              tunnel: w1336 -> [w1365]
              tunnel: w1334 -> [w1367]
              frame #0 {
                n363 = call <vilib>:"High Resolution Relative Seconds.vi"() -> ("relative seconds"=w1357:dbl)
              }
              frame #1 {
                n364 = Send Notification(notification=w1360, notifier=w1364, error in (no error)=w1363) -> (notifier out=w1361:refnum<notifier>, error out=w1362:errorcluster)
              }
              frame #2 {
                n365 = call <vilib>:"High Resolution Relative Seconds.vi"() -> ("relative seconds"=w1366:dbl)
              }
            }
            n366 = Subtract(x=w1342, y=w1341) -> (x-y=w1340:dbl)
            n367 = case shown="0" w1335 {
              tunnel: w1340 -> [_ w1355]
              tunnel: w1339 -> [w1352 w1354]
              tunnel: [w1352 w1353] -> w1338
              frame 0 {
              }
              frame 1, Default {
                n368 = Max & Min(x=w1355, y=w1354) -> (max(x,y)=w1353:dbl)  [unwired: 1 out]
              }
            }
          }
        }
        "Max Complexnote write" <- w1306
        n369 = while {
          tunnel: w1300 -> [w1322]
          tunnel: w1303 -> [w1323]
          tunnel: [w1320] -> _
          i -> [w1324]
          stop <- w1321 stop-if-true
          n370 = Bundle By Name(cluster=w1323, "Numeric"=w1324) -> ()  [unwired: 1 out]
          n371 = Wait on Notification(notifier=w1322, timeout in ms (-1)=0) -> (notification=w1320:T14, error out=w1321:errorcluster)  [unwired: 2 in, 2 out]
        }
        n372 = node-c288(w1317) -> ()  [unwired: 1 out]
        n373 = node-c288(w1315) -> ()  [unwired: 1 out]
        n374 = Subtract(x=w1314, y=w1313) -> (x-y=w1312:dbl)
        n375 = Divide(x=w1312, y=w1311) -> (x/y=w1308:dbl)
        "avg complexnote write" <- w1308
        n376 = Less?(x=w1306, y=4e-05) -> (x < y?=w1304:bool)
        n377 = Less?(x=w1308, y=5e-07) -> ()  [unwired: 1 out]
        n378 = Release Notifier(notifier=w1299, error in (no error)=w1298) -> (error out=w1297:errorcluster)  [unwired: 1 in, 2 out]
      }
      frame 1 {
        n379 = flat-sequence {
          tunnel: [w1429] -> w1413
          frame #0 {
            w1429 = FALSE ("stop")
            n380 = local write "stop"(w1429) -> ()
          }
        }
        n381 = node-c288() -> (w1428:T1)
        n382 = node-c288() -> (w1426:T1)
        n383 = timed-loop {
          timing: w1428 -> [_]
          timing-out: [_] -> w1427
          tunnel: w1412 -> [w1478]
          tunnel: [w1475] -> w1420
          tunnel: [w1473] -> w1424
          tunnel: [w1472] -> w1423
          tunnel: [w1471] -> w1421
          stop <- TRUE stop-if-true
          n384 = flat-sequence {
            tunnel: w1478 -> [w1480]
            tunnel: [w1480] -> w1476
            tunnel: [w1479] -> w1472
            tunnel: w1476 -> [w1483]
            tunnel: [w1482] -> w1474
            tunnel: [w1481] -> w1470
            tunnel: [w1488] -> w1475
            tunnel: w1474 -> [w1488]
            tunnel: [w1487] -> w1473
            tunnel: [w1486] -> w1471
            tunnel: w1470 -> [w1486]
            frame #0 {
              n385 = call <vilib>:"High Resolution Relative Seconds.vi"() -> ("relative seconds"=w1479:dbl)
            }
            frame #1 {
              w1481 = 10000
              n386 = for {
                N: w1481 -> [_]
                shift-right: [w1485] -> w1482
                shift-left: w1483 -> [w1485]
                shift-right: [w1484] -> _
                shift-left: _ -> [_]
                n387 = shared-variable ".\\variable Library.lvlib\\Variable1"() -> (w1484:T5)  [unwired: 1 in, 1 out]
              }
            }
            frame #2 {
              n388 = call <vilib>:"High Resolution Relative Seconds.vi"() -> ("relative seconds"=w1487:dbl)
            }
          }
        }
        n389 = timed-loop {
          timing: w1426 -> [_]
          timing-out: [_] -> w1425
          tunnel: w1420 -> [w1439]
          tunnel: [w1437] -> w1414
          tunnel: [w1434] -> w1417
          tunnel: [TRUE] -> w1411
          stop <- TRUE stop-if-true
          n390 = for {
            N: 100000 -> [_]
            shift-right: [w1450] -> w1437
            shift-left: w1439 -> [w1451]
            shift-right: [w1444] -> w1434
            shift-left: 0.0 -> [w1445]
            shift-right: [w1443] -> _
            shift-left: _ -> [w1449]
            i -> [w1441]
            n391 = flat-sequence {
              tunnel: w1451 -> [w1460]
              tunnel: [w1460] -> w1453
              tunnel: [w1459] -> w1447
              tunnel: w1449 -> [w1458]
              tunnel: [w1458] -> w1452
              tunnel: w1453 -> [w1462]
              tunnel: w1452 -> [_]
              tunnel: [w1461] -> w1442
              tunnel: [w1462] -> w1440
              tunnel: [w1465] -> w1450
              tunnel: [w1464] -> w1448
              tunnel: [w1463] -> w1443
              tunnel: w1442 -> [w1463]
              tunnel: w1440 -> [w1465]
              frame #0 {
                n392 = call <vilib>:"High Resolution Relative Seconds.vi"() -> ("relative seconds"=w1459:dbl)
              }
              frame #1 {
                n393 = shared-variable ".\\variable Library.lvlib\\Variable1"() -> (w1461:T5)  [unwired: 1 in, 1 out]
              }
              frame #2 {
                n394 = call <vilib>:"High Resolution Relative Seconds.vi"() -> ("relative seconds"=w1464:dbl)
              }
            }
            n395 = Subtract(x=w1448, y=w1447) -> (x-y=w1446:dbl)
            n396 = case shown="0" w1441 {
              tunnel: w1446 -> [_ w1457]
              tunnel: w1445 -> [w1454 w1456]
              tunnel: [w1454 w1455] -> w1444
              frame 0 {
              }
              frame 1, Default {
                n397 = Max & Min(x=w1457, y=w1456) -> (max(x,y)=w1455:dbl)  [unwired: 1 out]
              }
            }
          }
        }
        "Max raw local" <- w1417
        n398 = while {
          tunnel: w1413 -> [_]
          tunnel: w1412 -> [_]
          stop <- "stop" stop-if-true
          n399 = shared-variable ".\\variable Library.lvlib\\Variable1"(T5 {"State"=enum."Null", "Timing Statistics (us)"={"Period"={"Max"=0, "Min"=0}, "Wake Error"={"Max"=0, "Min"=0}, "Execute"={"Max"=0, "Min"=0}, "Housekeep"={"Max"=0, "Min"=0}, "Idle"={"Max"=0, "Min"=0}}, "FIFO Statistics (us)"={"From T0"={"Max"=0, "Min"=0}, "From Previous Plugin"={"Max"=0, "Min"=0}, "Output Error"={"Max"=0, "Min"=0}}, "error"={"status"=FALSE, "code"=0}, "Monitor Doubles"={"1"=0.0, "2"=0.0, "3"=0.0, "4"=0.0}, "Monitor U64"={"1"=0, "2"=0, "3"=0, "4"=0}, "Monitor I64"={"1"=0, "2"=0, "3"=0, "4"=0}, "Cleanup"={"Max"=0, "Min"=0}, "Create"=0, "Destroy"=0} ("Variable1")) -> ()  [unwired: 1 in, 1 out]
          n400 = Wait (ms)(milliseconds to wait=u32 0) -> ()  [unwired: 1 out]
        }
        n401 = node-c288(w1427) -> ()  [unwired: 1 out]
        n402 = node-c288(w1425) -> ()  [unwired: 1 out]
        n403 = Subtract(x=w1424, y=w1423) -> (x-y=w1422:dbl)
        n404 = local write "stop"(w1411) -> ()
        n405 = Divide(x=w1422, y=w1421) -> (x/y=w1419:dbl)
        "avg raw local" <- w1419
        n406 = Less?(x=w1417, y=9e-07) -> (x < y?=w1415:bool)
        n407 = Less?(x=w1419, y=5e-07) -> ()  [unwired: 1 out]
      }
    }
  }
  "error out" <- w4
  n408 = And Array Elements(Boolean array=w2) -> (logical AND=→"pass":bool)
